vi "bak.W7XBolo2018.vi"(1 "FPGA VI Reference In":refnum<k20>) -> (0 "FPGA VI Reference Out":refnum<k20>)   [LabVIEW 2014]
uses:
  <vilib>/Platform/TimedLoop/XDataNode/timing_clust.ctl
  <vilib>/Platform/TimedLoop/XDataNode/nitl_modes.ctl
  <vilib>/Platform/TimedLoop/XDataNode/wakeup.ctl
  <vilib>/userdefined/High Color/nirio_resource_hc.ctl
  <vilib>/FPGAPlugInAG/PCI-7813R/niLvFpga_Open_PCI-7813R.vi
  <vilib>/Utility/error.llb/Error Cluster From Error Code.vi
  <vilib>/rvi/errors/niLvFpgaAdjustHostInterfaceError.vi
  <vilib>/rvi/interface/common/niFpgaWaitOnOcc.vi
  <vilib>/httpClient/POSTBuffer.vi
  <vilib>/FPGAPlugInAG/PCI-7813R/niLvFpga_Close_PCI-7813R.vi
  <vilib>/rvi/interface/nirviOpenFPGA/nirviOpenFPGA.xnode
  FPGA Bitfiles/W7XBolo2017_FPGATarget_fmain2014_9xlV3GyHFfo.lvbitx
  f_main_2014.vi
  <vilib>/rvi/interface/nirviReadWriteControl/nirviReadWriteControl.xnode
  <vilib>/rvi/interface/nirviMethod/nirviMethod.xnode
  <vilib>/rvi/interface/nirviCloseFPGA/nirviCloseFPGA.xnode
  <vilib>/Platform/TimedLoop/XDataNode/XDataNode.xnode
  <vilib>/Platform/TimedLoop/XDataNode/XDNodeRunTimeDep.lvlib
  <vilib>/Analysis/NI_AALBase.lvlib
  <vilib>/httpClient/LabVIEWHTTPClient.lvlib
  <vilib>/Utility/file.llb/Read From Spreadsheet File (I64).vi
  <vilib>/Utility/file.llb/Read From Spreadsheet File (DBL).vi
  NiFpgaLv.dll
  <vilib>/DAQmx/configure/timing.llb/DAQmx Timing (Sample Clock).vi
  <vilib>/DAQmx/create/channels.llb/DAQmx Create Channel (AO-Voltage-Basic).vi
  <resource>/objmgr/daqmx.rc
  <vilib>/DAQmx/write.llb/DAQmx Write (Analog 1D DBL 1Chan NSamp).vi
  <vilib>/FPGAPlugInAG/PCI-7813R/niLvFpga_AcknowledgeIrq_PCI-7813R.vi
  <vilib>/FPGAPlugInAG/PCI-7813R/niLvFpga_ConfigureFifo_PCI-7813R.vi
  <vilib>/rvi/errors/niLvFpgaMergeErrorWithErrorCode.vi
panel:
  out "DAQ ready":bool
  out "DAQ wait time (should be = TWT":i32=-1
  in  "Pre-start time (ms) of DAQ \nTypically set to 1000 ms":i32=1000
  out "DAQ Timer":dbl
  in  "Tab Control 7":T1(tab)
  in  "Load from file":bool=TRUE
  in  "FreqSelRing":u16(ring) items=["0.8 ms", "1.6 ms", "3.2 ms", "6.4 ms", "12.8 ms", "19.2 ms"]
  in  "SecondFilter":bool=TRUE
  out "SampleTime":sgl=0.0004
  in  "Global or Individual DAC Settings\n\nIf global, dial on the right works.\nIf individual, enabled to either input manually via the array in IRS [Individual Range Settings] or load via file below.":bool caption="Range?"
  in  "DAC Range Setting":u8(knob)=3 scale=0.0..3.0
  in  "No. of Samples:":u32=10000
  out "Measured Time for DAQ [ms]\n \nShould rougly correspond to\nSampleTime * Samples":u32=8048
  in  "DAC settings file location":path=path "C:/LABVIEW/BLVFlo/LABVIEW/BLV/bolo_files/dac_settings.dat"
  in  "Trigger Source":i32(slide)=1 scale=0.0..2.0
  in  "Set Manual Time [ns]":i64=1503619200000000000
  out "Presamples \n(If -1, then no trigger detected)":i32
  in  "Wait-Time until Trigger\npublished on CODA\ntypically 10 s":u32=5000
  out "current epoch time timestamp":timestamp
  out "Number of nanoseconds with offset to 1904":i32
  out "Calibration Time":u32
  out "Countdown Time":u32
  out "Total wait time (TWT)\nTypically 59 s":u32
  in  "time before T1 = T0\nUsusally 60s":i32=60000
  in  "Tau00":dbl[](array[numeric])
  in  "Kappa00":dbl[](array[numeric])
  in  "RB000":dbl[](array[numeric])
  in  "Switch to fixed \nCalibration Values":bool
  in  "Clear all Values \nfrom Beginning":bool
  in  "Cancel Button":bool
  out "Actual Depth":u32=256
  out "T-Start [for Display)\nShould be -1 [s]":sgl=-1.0
  in  "Trigger No Choice\nfrom MDS+ Website\n0 for old\n1 during OP":i32
  in  "Tab Control":T2(tab)
  out "subvi timing":dbl
  out "rand plot sub":cluster{i32, "element":dbl}[](graph)
  in  "channel selection input":i32[][](array[numeric])
  out "kbolott_and_volume":dbl[][](array[numeric])
  in  "Read from file?":bool=TRUE
  in  "Path to kbolott and volume data file":path=path "C:/LABVIEW/BLVFlo/LABVIEW/BLV/bolo_files/kbolott_volume_all.dat"
  in  "Path to channel selection file":path=path "C:/LABVIEW/BLVFlo/LABVIEW/BLV/bolo_files/channel_selection.dat"
  in  "Read Channel Selection from file":bool=TRUE
  out "Channel Selection\nfrom input?":bool
  out "file import":i64[][](array[numeric])
  out "rand plot main":cluster{i32, "element":dbl}[](graph)
  out "sample array":i32[](array[numeric])
  out "cycle #":i32
  out "random array main":dbl[](array[numeric])
  out "rand array sub display":dbl[](array[numeric])
  out "timing average":dbl format="%.2f"
  out "final channel selection":i64[][](array[numeric])
  out "total\ntime":dbl
  out "pick-up cycle":i32
  out "subvi cycle #":dbl
  out "random array sub":dbl[](array[numeric])
  out "final channel\nselection size":i32
  in  "SubVI Test\nwith RAND array and\ntime measurement":bool
  out "Nsample array":i32[](array[numeric])
  out "real time p_rad":cluster{cluster{i32, dbl}[]}[](graph)
  out "RT P_rad":dbl[][](array[numeric])
  out "full power array":dbl[][](array[numeric])
  out "av power array":dbl[](array[numeric])
  out "final P_rad":dbl[](array[numeric])
  out "current P_rad sample":dbl format="%#_13g"
  in  "sample mode":i32(ring)=10123 items=["Finite Samples"=10178, "Continuous Samples"=10123, "Hardware Timed Single Point"=12522]
  in  "RegenMode":i32(ring)=10158 items=["Allow Regeneration"=10097, "Do Not Allow Regeneration"=10158]
  in  "rate of voltage sampling":dbl=100000.0 format="%#_13g"
  out "number of samples written on channel":u32
  in  "Stop Voltage Output":bool
  in  "maximum voltage @ 10MW":dbl=5.0 format="%#_13g"
  out "number of samples per iteration":dbl
  in  "Tab Control 4":enum32{"1 to 64", "65 to 128"}(tab)
  out "Raw 33-64":T3={"Channels 33 - 40"={"tstart"=-1.0, "FPGSampleTime"=0.0007999999797903001, array8x10000[80000 elements]}, "Channels 41 - 48"={"tstart"=-1.0, "FPGSampleTime"=0.0007999999797903001, array8x10000[80000 elements]}, "Channels 49 - 56"={"tstart"=-1.0, "FPGSampleTime"=0.0007999999797903001, array8x10000[80000 elements]}, "Channels 57 - 64"={"tstart"=-1.0, "FPGSampleTime"=0.0007999999797903001, array8x10000[80000 elements]}}
  out "Raw 1-32":T4={"Channels 1- 8"={"tstart"=-1.0, "FPGSampleTime"=0.0007999999797903001, array8x10000[80000 elements]}, "Channels 9 - 16"={"tstart"=-1.0, "FPGSampleTime"=0.0007999999797903001, array8x10000[80000 elements]}, "Channels 17 - 24"={"tstart"=-1.0, "FPGSampleTime"=0.0007999999797903001, array8x10000[80000 elements]}, "Channels 25 - 32"={"tstart"=-1.0, "FPGSampleTime"=0.0007999999797903001, array8x10000[80000 elements]}}
  out "Raw 97 - 128":T5
  out "Raw 65 - 97":T6={"Channels 65 - 71"={"tstart"=-1.0, "FPGSampleTime"=0.0007999999797903001, array8x10000[80000 elements]}, "Channels 73 - 80"={"tstart"=0.0, "FPGSampleTime"=0.0, []}, "Channels 81 - 88"={"tstart"=0.0, "FPGSampleTime"=0.0, []}, "Channels 89- 96"={"tstart"=0.0, "FPGSampleTime"=0.0, []}}
  in  "Tab Control 6":enum32{"1 to 64", "65 to 128"}(tab)=enum."65 to 128"
  out "Pow 33-64":T3
  out "Pow 1-32":T4={"Channels 1- 8"={"tstart"=-1.0, "FPGSampleTime"=0.0007999999797903001, array8x10000[80000 elements]}, "Channels 9 - 16"={"tstart"=-1.0, "FPGSampleTime"=0.0007999999797903001, array8x10000[80000 elements]}, "Channels 17 - 24"={"tstart"=0.0, "FPGSampleTime"=0.0, []}, "Channels 25 - 32"={"tstart"=0.0, "FPGSampleTime"=0.0, []}}
  out "Pow 97 - 128":T5
  out "Pow 65 - 96":T6={"Channels 65 - 71"={"tstart"=-1.0, "FPGSampleTime"=0.0007999999797903001, array8x10000[80000 elements]}, "Channels 73 - 80"={"tstart"=0.0, "FPGSampleTime"=0.0, []}, "Channels 81 - 88"={"tstart"=0.0, "FPGSampleTime"=0.0, []}, "Channels 89- 96"={"tstart"=0.0, "FPGSampleTime"=0.0, []}}
  out "Take file for DAC?":bool
  out "Take Input for DAC?":bool
  out "Range":u8[](array[numeric])
  out "DAC bits (range /1024)":u16[](array[numeric])
  out "full DAC\nfile input":i64[][](array[numeric])
  in  "input DAC settings":i64[](array[numeric])
  out "size(s)":i32
  out "DAC settings":i64[](array[numeric])
  in  "Tab Control 2":T7(tab)
  out "Offset 1-32":T4
  out "Offset 33-64":T3
  out "Offset 65 - 96":T6
  out "Offset 97 - 128":T5
  out "Mean (mV)":dbl[](array[numeric]) format="%10.6f"
  out "Peak to Peak \n      (microV)":dbl[](array[numeric]) format="%10.6f"
  out "StandardDeviation\n        (microV)":dbl[](array[numeric]) format="%10.7f"
  out "RefStatus 65-96":bool[](array[boolean])
  out "RefStatus 33-64":bool[](array[boolean])
  out "RefStatus 1-32":bool[](array[boolean])
  out "RefStatus 97-128":bool[](array[boolean])
  out "MessStatus 1-32":bool[](array[boolean])
  out "MessStatus 33-64":bool[](array[boolean])
  out "MessStatus 97-128":bool[](array[boolean])
  out "MessStatus 65-96":bool[](array[boolean])
  in  "Tab Control 5":T8(tab)
  out "MessCal 17-32":T9
  out "MessCal 1-16":T10
  out "MessCal 49 - 64":T11
  out "MessCal 33 - 49":T12
  out "MessCal 81 - 96":T13
  out "MessCal 65 - 80":T14
  out "MessCal 113 - 128":T15
  out "MessCal 97 - 112":T16
  out "RMESS":dbl[](array[numeric])
  out "KappaM":dbl[](array[numeric]) format="%10.4e"
  out "TauM":dbl[](array[numeric]) format="%10.4f"
  in  "Tab Control 3":T8(tab)=enum."97 to 128"
  out "RefCal 17-32":T9
  out "RefCal 1-16":T10
  out "RefCal 49 - 64":T11
  out "RefCal 33 - 48":T12
  out "RefCal 65 - 80":T14
  out "RefCal 81 - 96":T13
  out "RefCal 113 - 128":T15
  out "RefCal 97 - 112":T16
  out "TauR":dbl[](array[numeric]) caption="TauM" format="%10.4f"
  out "KappaR":dbl[](array[numeric]) format="%10.4e"
  out "RREF":dbl[](array[numeric])
  out "source":string
  out "code":i32
  out "status":bool
  out "Parlog error out":errorcluster
  out "Parlog error out  2":errorcluster
  out "error out":errorcluster
  out "Timed Out 2":bool
  out "Fehler":bool
  out "Fehler READ U+P":bool
  out "FilterTimeOut":bool
  out "result":bool
  out "headers chanDesc":string="HTTP/1.1 201 Created\r\nServer: Apache-Coyote/1.1\r\nLocation: http://archive-webapi.ipp-hgw.mpg.de/Test/raw/W7X/QSB_Bolometry/File_PARLOG/\r\nContent-Type: text/plain\r\nTransfer-Encoding: chunked\r\nDate: Wed, 15 Jul 2015 13:52:20 GMT\r\n\r\n"
  out "body chanDesc":string="Test/raw/W7X/QSB_Bolometry/File_PARLOG/ created."
  in  "chanDescs":T17(array[cluster])=[{"name"="HBCm_U30_01", "active"=1, "physicalQuantity"={"type"="A"}}, {"name"="HBCm_U30_02", "active"=1, "physicalQuantity"={"type"="A"}}, {"name"="HBCm_U30_03", "active"=1, "physicalQuantity"={"type"="A"}}, {"name"="HBCm_U30_04", "active"=1, "physicalQuantity"={"type"="A"}}, {"name"="HBCm_U30_05", "active"=1, "physicalQuantity"={"type"="A"}}, {"name"="HBCm_U30_06", "active"=1, "physicalQuantity"={"type"="A"}}, {"name"="HBCm_U30_07", "active"=1, "physicalQuantity"={"type"="A"}}, {"name"="HBCm_U30_08", "active"=1, "physicalQuantity"={"type"="A"}}, {"name"="HBCm_U30_09", "active"=1, "physicalQuantity"={"type"="A"}}, {"name"="HBCm_U30_10", "active"=1, "physicalQuantity"={"type"="A"}}, {"name"="HBCm_U30_11", "active"=1, "physicalQuantity"={"type"="A"}}, {"name"="HBCm_U30_12", "active"=1, "physicalQuantity"={"type"="A"}}, {"name"="HBCm_U30_013", "active"=1, "physicalQuantity"={"type"="A"}}, {"name"="HBCm_U30_14", "active"=1, "physicalQuantity"={"type"="A"}}, {"name"="HBCm_U30_15", "active"=1, "physicalQuantity"={"type"="A"}}, {"name"="HBCm_U30_16", "active"=1, "physicalQuantity"={"type"="A"}}, {"name"="HBCm_U30_17", "active"=1, "physicalQuantity"={"type"="A"}}, {"name"="HBCm_U30_18", "active"=1, "physicalQuantity"={"type"="A"}}, {"name"="HBCm_U30_19", "active"=1, "physicalQuantity"={"type"="A"}}, {"name"="HBCm_U30_20", "active"=1, "physicalQuantity"={"type"="A"}}, {"name"="HBCm_U30_21", "active"=1, "physicalQuantity"={"type"="A"}}, {"name"="HBCm_U30_22", "active"=1, "physicalQuantity"={"type"="A"}}, {"name"="HBCm_U30_23", "active"=1, "physicalQuantity"={"type"="A"}}, {"name"="HBCm_U30_24", "active"=1, "physicalQuantity"={"type"="A"}}, {"name"="HBCm_U30_25", "active"=1, "physicalQuantity"={"type"="A"}}, {"name"="HBCm_U30_26", "active"=1, "physicalQuantity"={"type"="A"}}, {"name"="HBCm_U30_27", "active"=1, "physicalQuantity"={"type"="A"}}, {"name"="HBCm_U30_28", "active"=1, "physicalQuantity"={"type"="A"}}, {"name"="HBCm_U30_29", "active"=1, "physicalQuantity"={"type"="A"}}, {"name"="HBCm_U30_30", "active"=1, "physicalQuantity"={"type"="A"}}, {"name"="HBCm_U30_31", "active"=1, "physicalQuantity"={"type"="A"}}, {"name"="HBCm_U30_32", "active"=1, "physicalQuantity"={"type"="A"}}, {"name"="VBCm_V21_01", "active"=1, "physicalQuantity"={"type"="A"}}, {"name"="VBCm_V21_02", "active"=1, "physicalQuantity"={"type"="A"}}, {"name"="VBCm_V21_03", "active"=1, "physicalQuantity"={"type"="A"}}, {"name"="VBCm_V21_04", "active"=1, "physicalQuantity"={"type"="A"}}, {"name"="VBCm_V21_05", "active"=1, "physicalQuantity"={"type"="A"}}, {"name"="VBCm_V21_06", "active"=1, "physicalQuantity"={"type"="A"}}, {"name"="VBCm_V21_07", "active"=1, "physicalQuantity"={"type"="A"}}, {"name"="VBCm_V21_08", "active"=1, "physicalQuantity"={"type"="A"}}, {"name"="VBCm_V21_09", "active"=1, "physicalQuantity"={"type"="A"}}, {"name"="VBCm_V21_10", "active"=1, "physicalQuantity"={"type"="A"}}, {"name"="VBCm_V21_11", "active"=1, "physicalQuantity"={"type"="A"}}, {"name"="VBCm_V21_12", "active"=1, "physicalQuantity"={"type"="A"}}, {"name"="VBCm_V21_13", "active"=1, "physicalQuantity"={"type"="A"}}, {"name"="VBCm_V21_14", "active"=1, "physicalQuantity"={"type"="A"}}, {"name"="VBCm_V21_15", "active"=1, "physicalQuantity"={"type"="A"}}, {"name"="VBCm_V21_16", "active"=1, "physicalQuantity"={"type"="A"}}, {"name"="VBCm_V21_17", "active"=1, "physicalQuantity"={"type"="A"}}, {"name"="VBCm_V21_18", "active"=1, "physicalQuantity"={"type"="A"}}, {"name"="VBCm_V21_19", "active"=1, "physicalQuantity"={"type"="A"}}, {"name"="VBCm_V21_20", "active"=1, "physicalQuantity"={"type"="A"}}, {"name"="VBCm_V21_21", "active"=1, "physicalQuantity"={"type"="A"}}, {"name"="VBCm_V21_22", "active"=1, "physicalQuantity"={"type"="A"}}, {"name"="VBCm_V21_23", "active"=1, "physicalQuantity"={"type"="A"}}, {"name"="VBCm_V21_24", "active"=1, "physicalQuantity"={"type"="A"}}, {"name"="VBCm_V21_25", "active"=1, "physicalQuantity"={"type"="A"}}, {"name"="VBCm_V21_26", "active"=1, "physicalQuantity"={"type"="A"}}, {"name"="VBCm_V21_27", "active"=1, "physicalQuantity"={"type"="A"}}, {"name"="VBCm_V21_28", "active"=1, "physicalQuantity"={"type"="A"}}, {"name"="VBCm_V21_29", "active"=1, "physicalQuantity"={"type"="A"}}, {"name"="VBCm_V21_30", "active"=1, "physicalQuantity"={"type"="A"}}, {"name"="VBCm_V21_31", "active"=1, "physicalQuantity"={"type"="A"}}, {"name"="VBCm_V21_32", "active"=1, "physicalQuantity"={"type"="A"}}, {"name"="VBCm_V21_33", "active"=1, "physicalQuantity"={"type"="A"}}, {"name"="VBCm_V21_34", "active"=1, "physicalQuantity"={"type"="A"}}, {"name"="VBCm_V21_35", "active"=1, "physicalQuantity"={"type"="A"}}, {"name"="VBCm_V21_36", "active"=1, "physicalQuantity"={"type"="A"}}, {"name"="VBCm_V21_37", "active"=1, "physicalQuantity"={"type"="A"}}, {"name"="VBCm_V21_38", "active"=1, "physicalQuantity"={"type"="A"}}, {"name"="VBCm_V21_39", "active"=1, "physicalQuantity"={"type"="A"}}, {"name"="VBCm_V21_40", "active"=1, "physicalQuantity"={"type"="A"}}, {"name"="VBCs_V21_01", "active"=1, "physicalQuantity"={"type"="A"}}, {"name"="VBCs_V21_02", "active"=1, "physicalQuantity"={"type"="A"}}, {"name"="VBCs_V21_03", "active"=1, "physicalQuantity"={"type"="A"}}, {"name"="VBCs_V21_04", "active"=1, "physicalQuantity"={"type"="A"}}, {"name"="VBCs_V21_05", "active"=1, "physicalQuantity"={"type"="A"}}, {"name"="VBCs_V21_06", "active"=1, "physicalQuantity"={"type"="A"}}, {"name"="VBCs_V21_07", "active"=1, "physicalQuantity"={"type"="A"}}, {"name"="VBCs_V21_08", "active"=1, "physicalQuantity"={"type"="A"}}, {"name"="HBCs_U30_01", "active"=1, "physicalQuantity"={"type"="A"}}, {"name"="HBCs_U30_02", "active"=1, "physicalQuantity"={"type"="A"}}, {"name"="HBCs_U30_03", "active"=1, "physicalQuantity"={"type"="A"}}, {"name"="HBCs_U30_04", "active"=1, "physicalQuantity"={"type"="A"}}, {"name"="HBCs_U30_05", "active"=1, "physicalQuantity"={"type"="A"}}, {"name"="HBCs_U30_06", "active"=1, "physicalQuantity"={"type"="A"}}, {"name"="HBCs_U30_07", "active"=1, "physicalQuantity"={"type"="A"}}, {"name"="HBCs_U30_08", "active"=1, "physicalQuantity"={"type"="A"}}, {"name"="HBCs_U30_09", "active"=1, "physicalQuantity"={"type"="A"}}, {"name"="HBCs_U30_10", "active"=1, "physicalQuantity"={"type"="A"}}, {"name"="HBCs_U30_11", "active"=1, "physicalQuantity"={"type"="A"}}, {"name"="HBCs_U30_12", "active"=1, "physicalQuantity"={"type"="A"}}, {"name"="HBCs_U30_13", "active"=1, "physicalQuantity"={"type"="A"}}, {"name"="HBCs_U30_14", "active"=1, "physicalQuantity"={"type"="A"}}, {"name"="HBCs_U30_15", "active"=1, "physicalQuantity"={"type"="A"}}, {"name"="HBCs_U30_16", "active"=1, "physicalQuantity"={"type"="A"}}]
  out "error out Cal":errorcluster
  out "parms error out":errorcluster
  in  "stop":bool
  out "Acquired Samples:":u32(slide) scale=-1.0..10000.0
  out "state":string="Wait for Start"
  # "If individual Range DAC Setting is selected, \nthe gain Range is loaded from following file:"
  # "Largest Offset ~ 20 mV\n40 mV Range should work \nfor all channels"
  # "Sample Rate Settings"
  # "FilterSelection"
  # "Set manual time [ns], epoch time"
  # "Get last trigger from http://sv-coda-wsvc-3/last_trigger"
  # "Get UTC Time not working"
  # "WENDELSTEIN - 7-X Bolometer DAQ System                                                                  v1.1.0"
  # "2018 @ P.Hacker"
  # "DAC Range shown for check:"
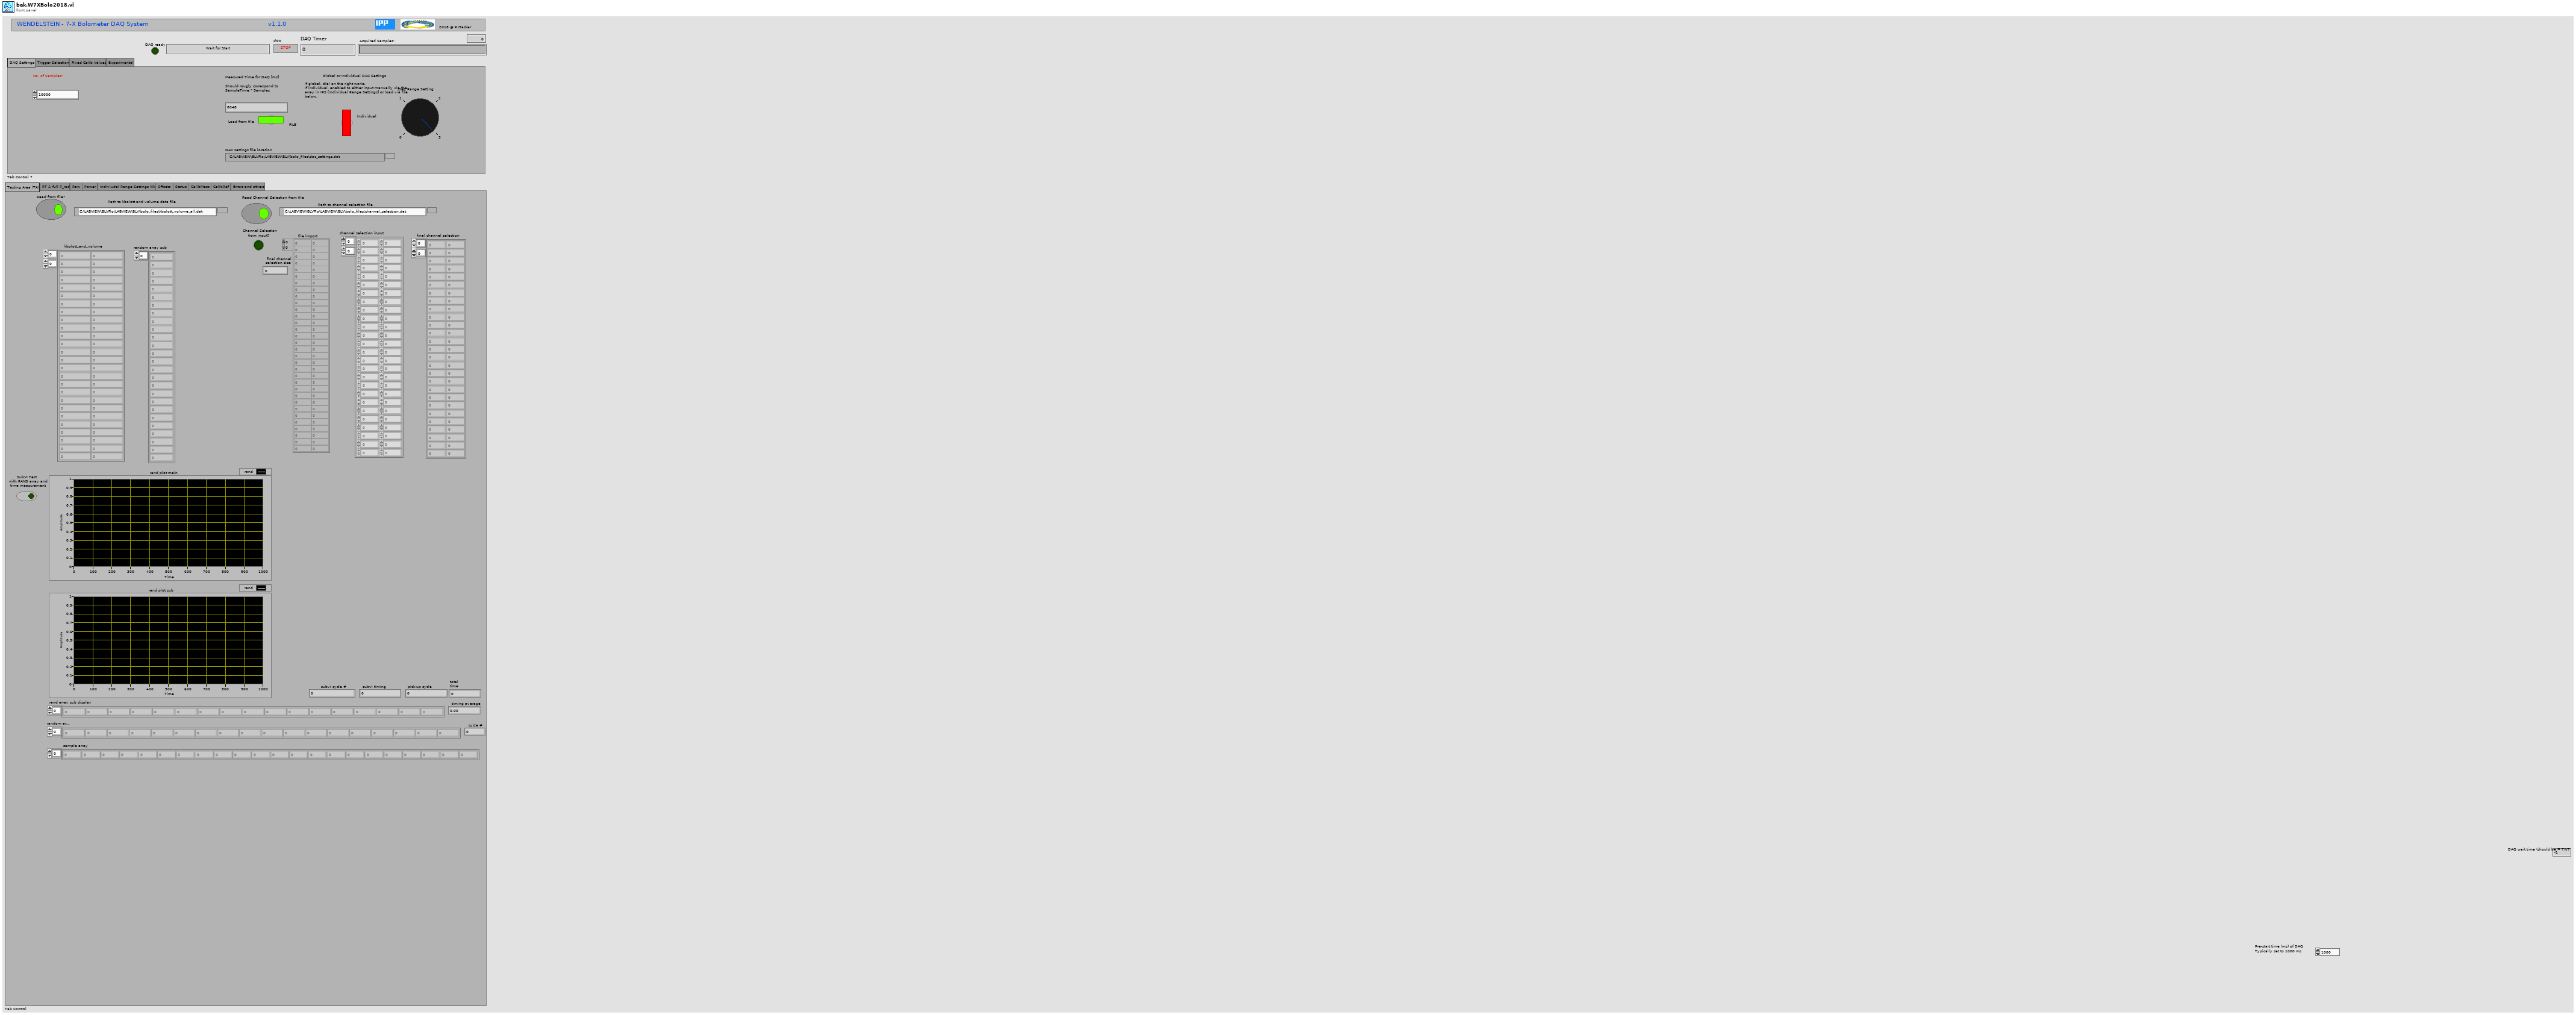
[diagram p1: front panel]
types:
  T1 = enum32{"DAQ Settings", "Trigger Selection", "Fixed Calib Values", "Experimental"}
  T2 = enum32{"Testing Area (TA)", "RT & full P_rad", "Raw", "Power", "Indiviudal Range Settings (IRS)", "Offsets", "Status", "CalibMess", "CalibRef", "Errors and others"}
  T3 = cluster{"Channels 33 - 40":cluster{"tstart":dbl, "FPGSampleTime":dbl, dbl[][]}, "Channels 41 - 48":cluster{"tstart":dbl, "FPGSampleTime":dbl, dbl[][]}, "Channels 49 - 56":cluster{"tstart":dbl, "FPGSampleTime":dbl, dbl[][]}, "Channels 57 - 64":cluster{"tstart":dbl, "FPGSampleTime":dbl, dbl[][]}}
  T4 = cluster{"Channels 1- 8":cluster{"tstart":dbl, "FPGSampleTime":dbl, dbl[][]}, "Channels 9 - 16":cluster{"tstart":dbl, "FPGSampleTime":dbl, dbl[][]}, "Channels 17 - 24":cluster{"tstart":dbl, "FPGSampleTime":dbl, dbl[][]}, "Channels 25 - 32":cluster{"tstart":dbl, "FPGSampleTime":dbl, dbl[][]}}
  T5 = cluster{"Channels 97 - 104":cluster{"tstart":dbl, "FPGSampleTime":dbl, dbl[][]}, "Channels 105 - 112":cluster{"tstart":dbl, "FPGSampleTime":dbl, dbl[][]}, "Channels 113 - 120":cluster{"tstart":dbl, "FPGSampleTime":dbl, dbl[][]}, "Channels 121 - 128":cluster{"tstart":dbl, "FPGSampleTime":dbl, dbl[][]}}
  T6 = cluster{"Channels 65 - 71":cluster{"tstart":dbl, "FPGSampleTime":dbl, dbl[][]}, "Channels 73 - 80":cluster{"tstart":dbl, "FPGSampleTime":dbl, dbl[][]}, "Channels 81 - 88":cluster{"tstart":dbl, "FPGSampleTime":dbl, dbl[][]}, "Channels 89- 96":cluster{"tstart":dbl, "FPGSampleTime":dbl, dbl[][]}}
  T7 = enum32{"1 to 32", "33 to 64", "65 to 96", "97 to128"}
  T8 = enum32{"1 to 32", "33 to 64", "65 to 96", "97 to 128"}
  T9 = cluster{"Channels 17 - 20":cluster{"tstart":sgl, "dt":sgl, "OutArray":dbl[][]}, "Channels 21 - 24":cluster{"tstart":sgl, "dt":sgl, "OutArray":dbl[][]}, "Channels 25 - 28":cluster{"tstart":sgl, "dt":sgl, "OutArray":dbl[][]}, "Channels 29 - 32":cluster{"tstart":sgl, "dt":sgl, "OutArray":dbl[][]}}
  T10 = cluster{"Channels 1- 4":cluster{"tstart":sgl, "dt":sgl, "OutArray":dbl[][]}, "Channels 5 - 8":cluster{"tstart":sgl, "dt":sgl, "OutArray":dbl[][]}, "Channels 9 - 12":cluster{"tstart":sgl, "dt":sgl, "OutArray":dbl[][]}, "Channels 13 - 16":cluster{"tstart":sgl, "dt":sgl, "OutArray":dbl[][]}}
  T11 = cluster{"Channels 49 - 52":cluster{"tstart":sgl, "dt":sgl, "OutArray":dbl[][]}, "Channels 53 - 56":cluster{"tstart":sgl, "dt":sgl, "OutArray":dbl[][]}, "Channels 57 - 60":cluster{"tstart":sgl, "dt":sgl, "OutArray":dbl[][]}, "Channels 61 - 64":cluster{"tstart":sgl, "dt":sgl, "OutArray":dbl[][]}}
  T12 = cluster{"Channels 33 - 36":cluster{"tstart":sgl, "dt":sgl, "OutArray":dbl[][]}, "Channels 37 - 40":cluster{"tstart":sgl, "dt":sgl, "OutArray":dbl[][]}, "Channels 41 - 44":cluster{"tstart":sgl, "dt":sgl, "OutArray":dbl[][]}, "Channels 45 - 48":cluster{"tstart":sgl, "dt":sgl, "OutArray":dbl[][]}}
  T13 = cluster{"Channels 81 - 84":cluster{"tstart":sgl, "dt":sgl, "OutArray":dbl[][]}, "Channels 85 - 88":cluster{"tstart":sgl, "dt":sgl, "OutArray":dbl[][]}, "Channels 89 - 92":cluster{"tstart":sgl, "dt":sgl, "OutArray":dbl[][]}, "Channels 93 - 96":cluster{"tstart":sgl, "dt":sgl, "OutArray":dbl[][]}}
  T14 = cluster{"Channels 65 - 68":cluster{"tstart":sgl, "dt":sgl, "OutArray":dbl[][]}, "Channels 69 - 72":cluster{"tstart":sgl, "dt":sgl, "OutArray":dbl[][]}, "Channels 73 - 76":cluster{"tstart":sgl, "dt":sgl, "OutArray":dbl[][]}, "Channels 77 - 80":cluster{"tstart":sgl, "dt":sgl, "OutArray":dbl[][]}}
  T15 = cluster{"Channels 113 - 116":cluster{"tstart":sgl, "dt":sgl, "OutArray":dbl[][]}, "Channels 117 - 120":cluster{"tstart":sgl, "dt":sgl, "OutArray":dbl[][]}, "Channels 121 - 124":cluster{"tstart":sgl, "dt":sgl, "OutArray":dbl[][]}, "Channels 125 - 128":cluster{"tstart":sgl, "dt":sgl, "OutArray":dbl[][]}}
  T16 = cluster{"Channels 97 - 100":cluster{"tstart":sgl, "dt":sgl, "OutArray":dbl[][]}, "Channels 101 - 104":cluster{"tstart":sgl, "dt":sgl, "OutArray":dbl[][]}, "Channels 104 - 108":cluster{"tstart":sgl, "dt":sgl, "OutArray":dbl[][]}, "Channels 109 - 112":cluster{"tstart":sgl, "dt":sgl, "OutArray":dbl[][]}}
  T17 = cluster{"name":string, "active":i32, "physicalQuantity":cluster{"type":string}}[]
  T18 = cluster{"Nchannel":i16, "ADCbits":i16, "BridgeVoltage (V)":sgl, "ExptSampleFrequency (Hz)":sgl, "CalibSampleFrequency (Hz)":sgl, "CalStep1 (V)":string, "CalStep2 (V)":string, "detector":string}[]
  T19 = cluster{"chanDescs":cluster{"name":string, "active":i32}[]}[]
  T20 = cluster{"tstart":sgl, "dt":sgl, "OutArray":dbl[][]}
  T21 = cluster{"Channels 9 - 12":cluster{"tstart":sgl, "dt":sgl, "OutArray":dbl[][]}, "Channels 9 - 12":cluster{"tstart":sgl, "dt":sgl, "OutArray":dbl[][]}, "Channels 9 - 12":cluster{"tstart":sgl, "dt":sgl, "OutArray":dbl[][]}, "Channels 9 - 12":cluster{"tstart":sgl, "dt":sgl, "OutArray":dbl[][]}}
  T22 = typedef "XDNodeRunTimeDep.lvlib/timing_clust.ctl" = cluster{"Expected End [f-1]":u64, "Actual End [f-1]":u64, "Finished Late? [f-1]":bool, "Expected End [i-1]":u64, "Actual End [i-1]":u64, "Finished Late? [i-1]":bool, "Expected Start [i]":u64, "Actual Start [i]":u64, "Expected Start [f]":u64, "Actual Start [f]":u64, "Source Name":string, "Structure Name":string, "Period":i64, "Deadline":i64, "Offset":i64, "Start":i64, "Priority":i32, "Timeout":i32, "Mode":T23, "Wakeup Reason":T24, "Error":errorcluster, "Source Type":string, "Secondary Source Type":string, "Global End Time":u64, "Global Start Time":u64, "Frame Duration":u64, "Iteration Duration":u64, "Assigned CPU":i32, "I/O Scan Engine Mode":u32}
  T23 = typedef "XDNodeRunTimeDep.lvlib/nitl_modes.ctl" = enum32{"No Change", "Process missed periods, maintain original phase", "Discard missed periods, maintain original phase", "Process missed periods, ignore original phase", "Discard missed periods, ignore original phase"}
  T24 = typedef "XDNodeRunTimeDep.lvlib/wakeup.ctl" = enum32{"Normal", "Aborted", "Asynchronous wakeup", "Timing source error", "Timed loop error", "Timeout"}
  T25 = typedef "nirio_resource_hc.ctl" = tag
  T26 = cluster{"Channels 33 - 40":cluster{"tstart":dbl, "FPGSampleTime":dbl, dbl[][]}, "Channels 41 - 48":cluster{"tstart":dbl, "FPGSampleTime":dbl, dbl[][]}, "Channels 49 - 56":cluster{"tstart":dbl, "FPGSampleTime":dbl, dbl[][]}, "Channels 57 - 58":cluster{"tstart":dbl, "FPGSampleTime":dbl, dbl[][]}}
  T27 = cluster{"Channels 1- 8":cluster{"tstart":sgl, "dt":sgl, "OutArray":dbl[][]}, "Channels 9 - 16":cluster{"tstart":sgl, "dt":sgl, "OutArray":dbl[][]}, "Channels 17 - 24":cluster{"tstart":sgl, "dt":sgl, "OutArray":dbl[][]}, "Channels 25 - 32":cluster{"tstart":sgl, "dt":sgl, "OutArray":dbl[][]}}
  T28 = cluster{"Channels 33 - 40":cluster{"tstart":sgl, "dt":sgl, "OutArray":dbl[][]}, "Channels 41 - 48":cluster{"tstart":sgl, "dt":sgl, "OutArray":dbl[][]}, "Channels 49 - 56":cluster{"tstart":sgl, "dt":sgl, "OutArray":dbl[][]}, "Channels 57 - 58":cluster{"tstart":sgl, "dt":sgl, "OutArray":dbl[][]}}
  T29 = typedef "LabVIEWHTTPClient.lvlib/ClientHandle.ctl" = refnum<k1>
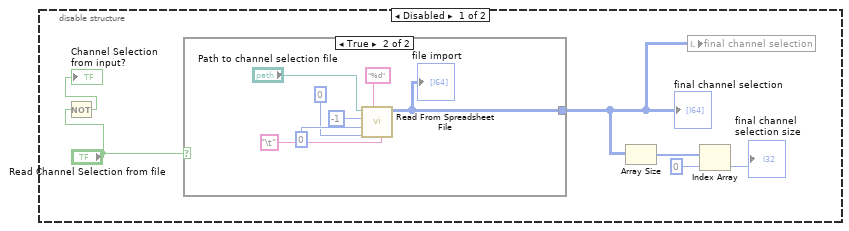
[diagram p5: hidden frame]
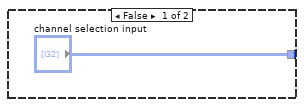
[diagram p6: hidden frame]
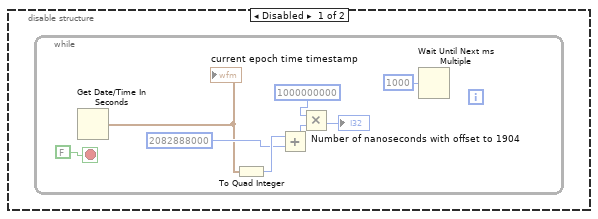
[diagram p7: hidden frame]
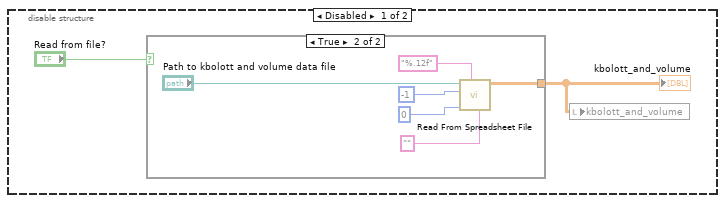
[diagram p8: hidden frame]
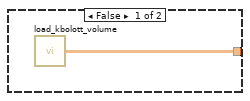
[diagram p9: hidden frame]
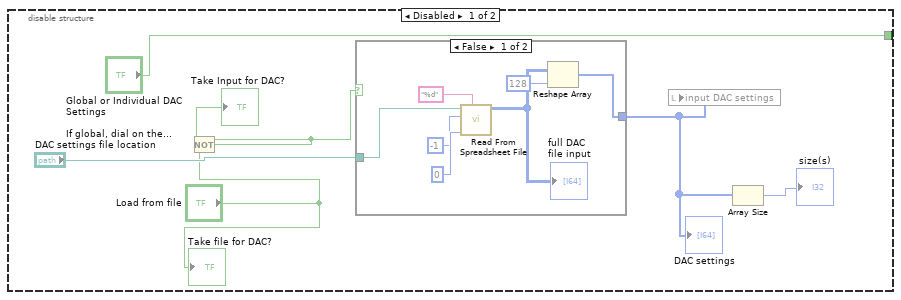
[diagram p10: hidden frame]
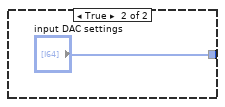
[diagram p11: hidden frame]
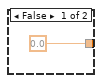
[diagram p14: hidden frame]
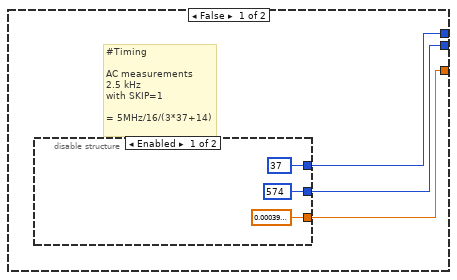
[diagram p17: hidden frame]
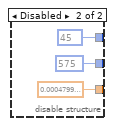
[diagram p18: hidden frame]
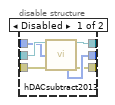
[diagram p19: hidden frame]
diagram:
  w4 = TRUE
  w9 = "W"  # Unit
  w20 = "Float"  # datatype
  w14 = "BoloPower"  # label
  w29 = i64 -1  # Time Array needs to be positive!
  w46 = i64 -1000000000  # Ns per Sec
  w77 = 1 ("sampleCount")
  w78 = 1 ("sampleCount")
  w81 = "s"  # Unit
  w102 = "V"  # Unit
  w106 = "A"  # Unit
  w26 = "A"  # Unit
  w110 = "A"  # Unit
  w117 = 1 ("sampleCount")
  w119 = 1 ("sampleCount")
  w121 = 1 ("sampleCount")
  w76 = 1 ("sampleCount")
  w49 = 1 ("sampleCount")
  w127 = "Float"  # datatype
  w97 = "mV"  # Unit
  w99 = "Offset"
  w133 = "Float"  # datatype
  w94 = "W"  # Unit
  w96 = "RKappa"  # label
  w135 = "Float"  # datatype
  w91 = "Ohms"  # Unit
  w93 = "RRes"  # label
  w137 = "Float"  # datatype
  w88 = "s"  # Unit
  w90 = "RTau"  # label
  w139 = "Float"  # datatype
  w85 = "W"  # Unit
  w87 = "MKappa"  # label
  w141 = "Float"  # datatype
  w84 = "Ohms"  # Unit
  w83 = "MRes"  # label
  w143 = "Float"  # datatype
  w80 = "MTau"  # label
  w50 = 10000 ("dimension size")
  w151 = 10000 ("sampleCount")
  w153 = "Float"  # datatype
  w112 = "A"  # Unit
  w114 = "BoloCalibRefFoilFit"  # label
  w154 = 10000 ("sampleCount")
  w156 = "Float"  # datatype
  w108 = "BoloCalibRefFoilCurrent"  # label
  w157 = 10000 ("sampleCount")
  w159 = "Float"  # datatype
  w6 = "BoloCalibMeasFoilFit"  # label
  w160 = 10000 ("sampleCount")
  w162 = "Float"  # datatype
  w104 = "BoloCalibMeasFoilCurrent"  # label
  w163 = "Float"  # datatype
  w101 = "BoloSignal"  # label
  # "I DONT KNOW ?!"
  # "channel selection routine for RT P_rad estimation"
  # "global switch for DAC settings and input relations, as well as ranges"
  # "import and load the kbolott and volume data for each camera/channel"
  # "time display for manual trigger and time stamp"
  # "SubVI, Reference and timeout test with basic tmp-VI"
  # "<< BoloCalibRefFoilFit <<"
  # "<< BoloCalibMeasFoilCurrent <<"
  # "<< BoloSignal <<"
  # ">> BoloReffFoilCurrent >>"
  # ">> BoloCalibMeasFoilFit >>"
  # ">> power >>"
  # "> power array >"
  # "> voltage array >"
  # "> voltage array >"
  # "> power >"
  # "Negative Sample Time [ns]"
  # "Time array for Bolo Signal"
  # "No of Samples DAQ"
  # "Time array for Bolo Signal"
  # "+ wait Time"
  # "-800000ns for 0.8ms"
  # "Negative Sample Time [ns]"
  # "Here Changed Names"
  # "Time Stamp for JSON Files"
  # "Sample rate for Calibration Arrays\n should be hardwired to calirbation settings"
  # "Sample Rate in [ns]"
  # "Calculated Start Time [ns]"
  # "NSample"
  # "10000"
  # "Initialize Array:\nDimesions Size = NSamples"
  # "Pulselength fixed for 0.4ms sample time and 10000 samples"
  # "NSamples * SampleTime = PulseLength"
  # "Data here is incorrect as well=!"
  # "Sample Time [s]\ncalculated to \nSample Time [ns]"
  # "Creating virtual Time Stamp\nfor Shot and for Calibration (Hardwired to 10000 samples)\nShot is depending on set sample rate"
  # "Index von dem Sample\nals der Trigger empfangen wurde"
  # "T1 Trigger\nkommt hier"
  # "A=> Internal full scale calibration\n8=> Internal zero scale calibration\nC=> System Zero scale Calibration\n2=> Continuous conversion\n\n5V reference\n80 mV scale\nChannel 1 input (voltage at bridge)\nMaster clock disable\n\np.15 7730 manual"
  # "AC 1.25 kHz Frequenz\nSKIP=0"
  n1 = flat-sequence {
    tunnel: [w207] -> w66
    tunnel: ["FPGA VI Reference In"] -> w70
    tunnel: [w208] -> w69
    tunnel: w66 -> [w208]
    frame #0 {
      n2 = Tick Count (ms)() -> (millisecond timer value=w207:u32)
    }
    frame #1 {
      n3 = case shown="True" "Clear all Values \nfrom Beginning" {
        frame False {
        }
        frame True {
          n4 = flat-sequence {
            frame #0 {
              w212 = bool[] [] ("MessStatus 1-32")
              w211 = dbl[] [] ("Kappa00")
              w214 = T20 {"tstart"=0.0, "dt"=0.0, "OutArray"=[]} ("Channels 9 - 12")
              # "Clear Graphs"
              n5 = local write "MessStatus 1-32"(w212) -> ()
              n6 = local write "RefStatus 97-128"(w212) -> ()
              n7 = local write "MessStatus 33-64"(w212) -> ()
              n8 = local write "MessStatus 65-96"(w212) -> ()
              n9 = local write "MessStatus 97-128"(w212) -> ()
              n10 = local write "RefStatus 1-32"(w212) -> ()
              n11 = local write "RefStatus 33-64"(w212) -> ()
              n12 = local write "RefStatus 65-96"(w212) -> ()
              n13 = local write "TauM"(w211) -> ()
              n14 = local write "TauR"(w211) -> ()
              n15 = local write "Tau00"(w211) -> ()
              n16 = local write "RMESS"(w211) -> ()
              n17 = local write "RREF"(w211) -> ()
              n18 = local write "RB000"(w211) -> ()
              n19 = Bundle("Channels 9 - 12"=w214, "Channels 9 - 12"=w214, "Channels 9 - 12"=w214, "Channels 9 - 12"=w214) -> (w213:T21)  [unwired: 1 in]
              n20 = local write "DAC bits (range /1024)"(w211) -> ()
              n21 = local write "MessCal 1-16"(w213) -> ()
              n22 = local write "MessCal 113 - 128"(w213) -> ()
              n23 = local write "MessCal 17-32"(w213) -> ()
              n24 = local write "MessCal 33 - 49"(w213) -> ()
              n25 = local write "Raw 65 - 97"(w213) -> ()
              n26 = local write "MessCal 49 - 64"(w213) -> ()
              n27 = local write "Raw 97 - 128"(w213) -> ()
              n28 = local write "MessCal 65 - 80"(w213) -> ()
              n29 = local write "MessCal 81 - 96"(w213) -> ()
              n30 = local write "MessCal 97 - 112"(w213) -> ()
              n31 = local write "RefCal 1-16"(w213) -> ()
              n32 = local write "RefCal 113 - 128"(w213) -> ()
              n33 = local write "Raw 1-32"(w213) -> ()
              n34 = local write "Raw 33-64"(w213) -> ()
              n35 = local write "RefCal 33 - 48"(w213) -> ()
              n36 = local write "Pow 1-32"(w213) -> ()
              n37 = local write "RefCal 49 - 64"(w213) -> ()
              n38 = local write "Pow 33-64"(w213) -> ()
              n39 = local write "RefCal 65 - 80"(w213) -> ()
              n40 = local write "Offset 1-32"(w213) -> ()
              n41 = local write "RefCal 81 - 96"(w213) -> ()
              n42 = local write "Offset 33-64"(w213) -> ()
              n43 = local write "RefCal 97 - 112"(w213) -> ()
              n44 = local write "Offset 65 - 96"(w213) -> ()
              n45 = local write "Offset 97 - 128"(w213) -> ()
              n46 = local write "Pow 65 - 96"(w213) -> ()
              n47 = local write "RefCal 17-32"(w213) -> ()
              n48 = local write "Pow 97 - 128"(w213) -> ()
              n49 = local write "KappaR"(w211) -> ()
              n50 = local write "Peak to Peak \n      (microV)"(w211) -> ()
              n51 = local write "Mean (mV)"(w211) -> ()
              n52 = local write "Kappa00"(w211) -> ()
              n53 = local write "StandardDeviation\n        (microV)"(w211) -> ()
              n54 = local write "KappaM"(w211) -> ()
              n55 = local write "Range"(w211) -> ()
            }
          }
        }
      }
    }
  }
  n56 = disable-structure shown="Disabled" {
    frame Disabled {
      n57 = case shown="True" "SubVI Test\nwith RAND array and\ntime measurement" {
        frame False {
        }
        frame True {
          n58 = flat-sequence {
            tunnel: [w220] -> w217
            tunnel: [w219] -> w216
            tunnel: w217 -> [w235]
            tunnel: w216 -> [w229]
            frame #0 {
              w219 = 1000 ("x")
              n59 = Initialize Array(0, w219) -> (w224:i32[])
              n60 = for {
                N: w219 -> [_]
                shift-right: [w225] -> w220
                shift-left: w224 -> [w227]
                i -> [w226]
                n61 = Replace Array Subset(array=w227, new element=w226, index=w226) -> (w225:i32[])
              }
              "sample array" <- w220
              n62 = local write "state"("pre-occupying test arrays" ("state")) -> ()
              n63 = Initialize Array(0.0 ("element"), w219) -> (w218:dbl[])
              "random array main" <- w218
              "random array sub" <- w218
              n64 = local write "random array main"(w218) -> ()
              n65 = local write "random array sub"(w218) -> ()
            }
            frame #1 {
              # "testing for array output"
              n66 = call <vilib>:"High Resolution Relative Seconds.vi"() -> ("relative seconds"=w231:dbl)
              n67 = control-ref of="rand array sub display"() -> (w233:refnum<vi>)
              n68 = local read "No. of Samples:"() -> (w228:u32)
              n69 = for {
                N: w228 -> [_]
                i -> [w241]
                n70 = local read "av power array"() -> (w245:dbl[])
                n71 = local read "final P_rad"() -> (w242:dbl[])
                n72 = Random Number (0-1)() -> (number: 0 to 1=w244:dbl)
                n73 = Replace Array Subset(array=w245, new element=w244, index=w241) -> (w243:dbl[])
                n74 = Random Number (0-1)() -> (number: 0 to 1=w240:dbl)
                n75 = Replace Array Subset(array=w242, new element=w240, index=w241) -> (w239:dbl[])
                n76 = local write "av power array"(w243) -> ()
                n77 = local write "final P_rad"(w239) -> ()
                n78 = Wait Until Next ms Multiple(millisecond multiple=u32 50) -> ()  [unwired: 1 out]
              }
              n79 = control-ref of="subvi cycle #"() -> (w230:refnum<vi>)
              n80 = control-ref of="subvi timing"() -> (w232:refnum<vi>)
              n81 = for {
                N: w229 -> [_]
                tunnel: w235 -> [w258]
                i -> [w259]
                n82 = local read "random array main"() -> (w257:dbl[])
                n83 = Wait Until Next ms Multiple(millisecond multiple=10) -> ()  [unwired: 1 out]
                n84 = Random Number (0-1)() -> (number: 0 to 1=w261:dbl)
                n85 = Replace Array Subset(array=w257, new element=w261, index=w259) -> (w256:dbl[])
                n86 = Build Cluster Array(w258, w256) -> (→"rand plot main":cluster{i32, "element":dbl}[])
                n87 = local write "random array main"(w256) -> ()
                "cycle #" <- w259
              }
              n88 = local read "random array sub"() -> (w234:dbl[])
              n89 = control-ref of="rand plot sub"() -> (w236:refnum<vi>)
              n90 = local write "state"("subvi and real time plot" ("state")) -> ()
              n91 = call "test.vi"("length"=w229, "subvi cycle"=w230, "sample array"=w235, "rand array sub"=w234, "subvi timing"=w232, "Graph Refnum"=w236, "start time"=w231, "rand array sub refnum"=w233) -> ()  [unwired: 4 in]
              n92 = while {
                tunnel: w231 -> [w253]
                tunnel: w229 -> [w247]
                i -> [w249]
                stop <- w254 stop-if-true
                n93 = Multiply(x=w247, y=10) -> (x*y=w248:i32)
                n94 = call <vilib>:"High Resolution Relative Seconds.vi"() -> ("relative seconds"=w252:dbl)
                n95 = Greater?(x=w248, y=w249) -> (0:w254:bool)
                n96 = Subtract(x=w252, y=w253) -> (x-y=w251:dbl)
                "total\ntime" <- w251
                n97 = Divide(x=w251, y=w249) -> (x/y=→"timing average":dbl)
                n98 = Wait Until Next ms Multiple(millisecond multiple=1) -> ()  [unwired: 1 out]
                "pick-up cycle" <- w249
              }
            }
          }
        }
      }
    }
    frame Enabled {
    }
  }
  n99 = Not A Number/Path/Refnum?(number/path/refnum=w70) -> (NaN/Path/Refnum?=w1:bool)
  n100 = disable-structure shown="Enabled" {
    frame Enabled {
      n101 = flat-sequence {
        tunnel: "Cancel" ("name (unnamed)") -> [w292]
        tunnel: "Transferred1" ("name (unnamed)") -> [w291]
        tunnel: u32 0 -> [w290]
        tunnel: FALSE -> [w289]
        tunnel: [w288] -> w271
        tunnel: [w287] -> w270
        tunnel: [w286] -> w269
        tunnel: [w285] -> w268
        tunnel: [u32 0] -> w263
        frame #0 {
          n102 = local write "stop"(FALSE ("stop")) -> ()
          n103 = RT FIFO Create(0:w291, 1:w290) -> (8:w285:refnum<k33>, 11:w286:errorcluster)  [unwired: 2 in, 5 out]
          n104 = RT FIFO Create(0:w292, 1:w289) -> (8:w288:refnum<k33>, 11:w287:errorcluster)  [unwired: 3 in, 4 out]
        }
      }
      n105 = node-c288() -> (w277:T22)  [unwired: 1 in, 4 out]
      n106 = timed-loop {
        tunnel: w271 -> [w303]
        tunnel: w270 -> [w302]
        tunnel: w269 -> [w301]
        tunnel: w268 -> [w300]
        shift-right: [w299] -> _
        shift-left: w263 -> [w293]
        tunnel: [w298] -> w265
        tunnel: [w297] -> w264
        tunnel: [w296] -> w267
        tunnel: [w295] -> w266
        timing: w277 -> [_]
        timing-out: [_] -> w276
        stop <- "stop" stop-if-true
        n107 = RT FIFO Read(0:w300, 1:w293, 3:w301) -> (8:w296:refnum<k33>, 9:w299:u32, 11:w295:errorcluster)  [unwired: 3 out]
        n108 = RT FIFO Write(0:w303, 1:"Cancel Button", 3:w302) -> (8:w298:refnum<k33>, 11:w297:errorcluster)  [unwired: 1 in, 3 out]
        "Acquired Samples:" <- w293
      }
      n109 = node-c288(w276) -> ()  [unwired: 1 out]
      n110 = flat-sequence {
        tunnel: w267 -> [w282]
        tunnel: w266 -> [w281]
        tunnel: w265 -> [w280]
        tunnel: w264 -> [w279]
        frame #0 {
          n111 = RT FIFO Delete(0:w282, 3:w281) -> ()  [unwired: 1 in, 1 out]
          n112 = RT FIFO Delete(0:w280, 3:w279) -> ()  [unwired: 1 in, 1 out]
          n113 = local write "stop"(FALSE ("stop")) -> ()
        }
      }
    }
    frame Disabled {
    }
  }
  n114 = disable-structure shown="Enabled" {
    frame Disabled {
      n115 = while {
        stop <- FALSE stop-if-true
        n116 = Get Date/Time In Seconds() -> (seconds since 1Jan1904=w314:timestamp)
        "current epoch time timestamp" <- w314
        n117 = To Quad Integer(1:w314) -> (0:w316:i64)
        n118 = Add(x=w316, y=2082888000) -> (x+y=w310:i64)
        n119 = Multiply(x=1000000000, y=w310) -> (x*y=→"Number of nanoseconds with offset to 1904":i64)
        n120 = Wait Until Next ms Multiple(millisecond multiple=1000) -> ()  [unwired: 1 out]
      }
    }
    frame Enabled {
    }
  }
  n121 = disable-structure shown="Enabled" {
    frame Disabled {
      n122 = case shown="True" "Read from file?" {
        tunnel: [w319 w320] -> w317
        frame False {
          n123 = call "load_kbolott_volume.vi"() -> ("output"=w319:dbl[][])
        }
        frame True {
          n124 = call-poly <vilib>:"Read From Spreadsheet File.vi"("delimiter (\\t)"="" ("delimiter (\\t)"), "format (%.3f)"="%.12f", "max characters/row  (no limit:0)"=0, "number of rows (all:-1)"=-1, "file path (dialog if empty)"="Path to kbolott and volume data file") -> ("all rows"=w320:dbl[][])  [unwired: 2 in, 4 out]
        }
      }
      "kbolott_and_volume" <- w317
      n125 = local write "kbolott_and_volume"(w317) -> ()
    }
    frame Enabled {
    }
  }
  n126 = disable-structure shown="Enabled" {
    disable-tunnel: ["Global or Individual DAC Settings\n\nIf global, dial on the right works.\nIf individual, enabled to either input manually via the array in IRS [Individual Range Settings] or load via file below." _] -> w3
    frame Disabled {
      n127 = Not(x="Load from file") -> (.not. x?=w329:bool)
      "Take Input for DAC?" <- w329
      n128 = case shown="False" w329 {
        tunnel: "DAC settings file location" -> [w338 _]
        tunnel: [w332 "input DAC settings"] -> w326
        frame False {
          n129 = call-poly <vilib>:"Read From Spreadsheet File.vi"("format (%d)"="%d", "max characters/row  (no limit:0)"=0, "number of rows (all:-1)"=-1, "file path (dialog if empty)"=w338) -> ("all rows"=w333:i64[][])  [unwired: 3 in, 4 out]
          "full DAC\nfile input" <- w333
          n130 = Reshape Array(w333, 128 ("dimension size")) -> (w332:i64[])
        }
        frame True {
        }
      }
      "DAC settings" <- w326
      n131 = local write "input DAC settings"(w326) -> ()
      n132 = Array Size(array=w326) -> (size(s)=→"size(s)":i32)
      "Take file for DAC?" <- "Load from file"
    }
    frame Enabled {
    }
  }
  n133 = disable-structure shown="Enabled" {
    frame Disabled {
      n134 = Not(x="Read Channel Selection from file") -> (.not. x?=→"Channel Selection\nfrom input?":bool)
      n135 = case shown="True" "Read Channel Selection from file" {
        tunnel: ["channel selection input" w347] -> w343
        frame False {
        }
        frame True {
          n136 = call-poly <vilib>:"Read From Spreadsheet File.vi"("delimiter (\\t)"="\t" ("delimiter (\\t)"), "format (%d)"="%d", "max characters/row  (no limit:0)"=0, "start of read offset (chars.:0)"=0, "number of rows (all:-1)"=-1, "file path (dialog if empty)"="Path to channel selection file") -> ("all rows"=w347:i64[][])  [unwired: 1 in, 4 out]
          "file import" <- w347
        }
      }
      "final channel selection" <- w343
      n137 = Array Size(array=w343) -> (size(s)=w342:i32[])
      n138 = local write "final channel selection"(w343) -> ()
      n139 = Index Array(array=w342, index=0) -> (element=→"final channel\nselection size":i32)
    }
    frame Enabled {
    }
  }
  n140 = case shown="True" w1 {
    tunnel: [w354 w356] -> w180
    tunnel: [_ w355] -> w179
    tunnel: w70 -> [w354 _]
    frame False {
    }
    frame True {
      n141 = xnode "Open FPGA VI Reference"("resource name"=T25 "RIO0") -> ("FPGA VI Reference Out"=w356:refnum<k20>, "error out"=w355:errorcluster)  [unwired: 1 in]
    }
  }
  "error out" <- w179
  n142 = xnode "Read/Write Control"("FPGA VI Reference In"=w180, "error in"=w179, "cancel"=TRUE ("clrFifo"), "Test"=FALSE) -> ("FPGA VI Reference Out"=w206:refnum<k20>, "error out"=w205:errorcluster)
  n143 = flat-sequence {
    tunnel: w206 -> [w364]
    tunnel: w205 -> [w363]
    tunnel: [w362] -> w204
    tunnel: [w361] -> w203
    frame #0 {
      n144 = Wait (ms)(milliseconds to wait=u32 100) -> ()  [unwired: 1 out]
      n145 = xnode "Invoke Method"("FPGA VI Reference In"=w364, "error in"=w363, "IRQ Number(s)"=i32[] [0, 1, 2, 3]) -> ("FPGA VI Reference Out"=w362:refnum<k20>, "error out"=w361:errorcluster)
      "state" <- "Start (100 ms)" ("state")
    }
  }
  n146 = flat-sequence {
    tunnel: w203 -> [w366]
    tunnel: [w365] -> w199
    tunnel: w204 -> [w367]
    tunnel: [w368] -> w182
    frame #0 {
      n147 = call "hReset2014.vi"("error in"=w366, "FPGA VI Reference In"=w367) -> ("error out"=w365:errorcluster, "FPGA VI Reference Out"=w368:refnum<k20>)  [unwired: 4 in]
      n148 = local write "state"("Reset" ("state")) -> ()
    }
  }
  n149 = call "hFilterReg2014.vi"("error in"=w199, "Filter Modus"=u16 61 ("t"), "Frequenz"=u8 79 ("AC 1kHz Frequenz\nSKIP=0"), "FPGA VI Reference In"=w182) -> ("error out"=w184:errorcluster, "Timed Out"=w193:bool, "FPGA VI Reference Out"=w183:refnum<k20>)  [unwired: 1 in]
  "FilterTimeOut" <- w193
  n150 = call "hModeReg2014.vi"("error in"=w184, "Mode"=u16 41144, "FPGA VI Reference In"=w183) -> ("error out"=w187:errorcluster, "Timeout"=w197:bool, "FPGA VI Reference Out"=w190:refnum<k20>)  [unwired: 2 in]
  n151 = call "hModeReg2014.vi"("error in"=w187, "Mode"=u16 32952, "FPGA VI Reference In"=w190) -> ("error out"=w186:errorcluster, "Timeout"=w198:bool, "FPGA VI Reference Out"=w189:refnum<k20>)  [unwired: 2 in]
  n152 = call "hModeReg2014.vi"("error in"=w186, "Mode"=u16 8376, "FPGA VI Reference In"=w189) -> ("error out"=w195:errorcluster, "Timeout"=w196:bool, "FPGA VI Reference Out"=w194:refnum<k20>)  [unwired: 2 in]
  n153 = Compound Arithmetic op=OR(w197, w198, w196, w193) -> (→"DAQ ready":bool)
  n154 = case shown="False" w4 {
    tunnel: [w396 w911] -> w67
    tunnel: [w395 w910] -> w202
    tunnel: w194 -> [w555 w911]
    tunnel: w195 -> [w554 w910]
    tunnel: [w415 _] -> w22
    tunnel: [w450 _] -> w149
    tunnel: [w445 _] -> w150
    tunnel: [w441 _] -> w147
    tunnel: [w438 _] -> w148
    tunnel: [w393 _] -> w71
    tunnel: [w436 _] -> w132
    tunnel: [w381 _] -> w72
    tunnel: [w435 _] -> w131
    tunnel: [w434 _] -> w130
    tunnel: [w413 _] -> w129
    tunnel: [w417 _] -> w30
    tunnel: w69 -> [w386 _]
    tunnel: [w383 _] -> w23
    tunnel: [w374 _] -> w21
    tunnel: w3 -> [w373 _]
    frame False {
      w456 = 2000
      w469 = u8 125  # Frequenz
      w514 = 0.0008 ("FPGSampleTime")
      w509 = 0.0
      w380 = 40.0  # Rcable
      w549 = 10.0  # Rload
      w568 = sgl 0.0004  # dt
      w569 = sgl 0.0  # tstart
      w572 = sgl 0.0004  # dt
      w573 = sgl 0.0  # tstart
      w577 = sgl 80.0 ("Scale(mV)")
      # "> voltage array >"
      # "> power >"
      # "> voltage array >"
      # "Offset Shift manually disabled because not need for low power discharges"
      # "Absolute Timer [ms] (Now)\n-\nAbsolute Timer [ms] (At Start)\n=\nTime need until start of DAQ"
      # "Startzeit - 14 s"
      # "old time from OP1"
      # "Store raw data"
      # "#Timing \n\nAC measurements\n2.083 kHz\nwith SKIP=1 \n\n= 5MHz/16/(3*45+15)"
      # "#Offset measurement"
      # "#Offset applied"
      # "#Range for measurements"
      # "A=> Internal full scale calibration\n8=> Internal zero scale calibration\nC=> System Zero scale Calibration\n2=> Continuous conversion\n\n2.5V reference\n80 mV scale\nChannel 2 input (voltage at shunt)\nMaster clock disable\n\np.15 7730 manual"
      n155 = local read "DAC settings"() -> (w372:i64[])
      n156 = flat-sequence {
        tunnel: [w715] -> w391
        tunnel: [w714] -> w390
        tunnel: w555 -> [w718]
        tunnel: w554 -> [w717]
        tunnel: w456 -> [w723]
        tunnel: [w722] -> w458
        tunnel: w391 -> [w725]
        tunnel: w390 -> [w724]
        tunnel: [w721] -> w457
        tunnel: [w731] -> w633
        tunnel: [w730] -> w632
        tunnel: [w729] -> w630
        tunnel: w456 -> [w727]
        tunnel: w458 -> [w733]
        tunnel: w457 -> [w732]
        frame #0 {
          n157 = call "hComRegStart2013.vi"("error in"=w717, "FPGA VI Reference In"=w718) -> ("error out"=w714:errorcluster, "Timed Out"=→"Timed Out 2":bool, "FPGA VI Reference Out"=w715:refnum<k20>)  [unwired: 3 in]
          n158 = call "Wait3"("Count(mSec)"=u32 3000) -> ()  [unwired: 1 out]
        }
        frame #1 {
          n159 = call "Wait6"("Count(mSec)"=u32 1000) -> ()  [unwired: 1 out]
          n160 = local write "state"("SyncRun (1000 ms)" ("state")) -> ()
          n161 = call "hSync&StartSampling2013.vi"("error in"=w724, "#Samples"=w723, "FPGA VI Reference In"=w725) -> ("error out"=w722:errorcluster, "FPGA VI Reference Out"=w721:refnum<k20>)  [unwired: 1 in]
        }
        frame #2 {
          n162 = call "hReadChannelsRTDMA2013.vi"("FPGA VI Reference In"=w732, "Nsamples"=w727, "error in"=w733) -> ("FPGA VI Reference Out"=w731:refnum<k20>, "Fehler"=→"Fehler":bool, "RawArray"=w729:i16[][], "error out"=w730:errorcluster)  [unwired: 2 in]
          n163 = local write "state"("ReadOffset" ("state")) -> ()
        }
      }
      n164 = property on="Acquired Samples:" class="Slide (strict)"("Scale.Range:Maximum"=w456) -> ()  [unwired: 2 in, 2 out]
      n165 = call "hSoftReset2013.vi"("error in"=w632, "FPGA VI Reference In"=w633) -> ("error out"=w467:errorcluster, "FPGA VI Reference Out"=w460:refnum<k20>)  [unwired: 4 in]
      n166 = call "Int2Volt2D.vi"("IntegerArray"=w630, "Scale(mV)"=sgl 80.0) -> ("RealArray"=w505:sgl[][])
      n167 = xnode "Read/Write Control"("FPGA VI Reference In"=w460, "error in"=w467, "HIREF"=TRUE) -> ("FPGA VI Reference Out"=w463:refnum<k20>, "error out"=w462:errorcluster)
      n168 = for {
        tunnel: w505 -> [w754] mode=indexing
        tunnel: [w753] -> w502 mode=indexing
        tunnel: [w752] -> w504 mode=indexing
        tunnel: [w751] -> w503 mode=indexing
        n169 = Array Subset(array=w754, index=500, length=1000) -> (w756:sgl[])
        n170 = call <vilib>:"Std Deviation and Variance.vi"("X"=w756, "Weighting (Sample)"=enum16{"Sample", "Population"}."Population") -> ("mean"=w752:dbl, "standard deviation"=w751:dbl)  [unwired: 1 out]
        n171 = Array Max & Min(array=w756) -> (max value=w759:sgl, min value=w760:sgl)  [unwired: 2 out]
        n172 = Subtract(x=w759, y=w760) -> (x-y=w753:sgl)
      }
      n173 = Array Subset(array=w505, index (row)=0, length (row)=64, index (col)=0) -> (w519:sgl[][])  [unwired: 1 in]
      n174 = Array Subset(array=w505, index (row)=64, length (row)=64, index (col)=0) -> (w515:sgl[][])  [unwired: 1 in]
      n175 = call "Visualize_Signals64.vi"("FPGSampleTime"=w514, "tstart"=w509, "Signals"=w519) -> ("plot(Signals) 33-64"=→"Offset 33-64":T26, "plot(Signals) 1-32"=→"Offset 1-32":T4)  [unwired: 7 in]
      n176 = call "Visualize_Signals64.vi"("FPGSampleTime"=w514, "tstart"=w509, "Signals"=w515) -> ("plot(Signals) 33-64"=→"Offset 97 - 128":T26, "plot(Signals) 1-32"=→"Offset 65 - 96":T4)  [unwired: 7 in]
      n177 = call "hFilterReg2014.vi"("error in"=w462, "Filter Modus"=u16 512 ("t"), "Frequenz"=w469, "FPGA VI Reference In"=w463) -> ("error out"=w461:errorcluster, "FPGA VI Reference Out"=w464:refnum<k20>)  [unwired: 1 in, 1 out]
      n178 = call "hModeReg2014.vi"("error in"=w461, "Mode"=u16 41017, "FPGA VI Reference In"=w464) -> ("error out"=w473:errorcluster, "FPGA VI Reference Out"=w472:refnum<k20>)  [unwired: 2 in, 1 out]
      n179 = call "hModeReg2014.vi"("error in"=w473, "Mode"=u16 32825, "FPGA VI Reference In"=w472) -> ("error out"=w470:errorcluster, "FPGA VI Reference Out"=w471:refnum<k20>)  [unwired: 2 in, 1 out]
      n180 = Multiply(x=w504, y=1000.0 ("Scale")) -> (x*y=w417:dbl[])
      "Mean (mV)" <- w417
      n181 = Multiply(x=w503, y=1000000.0 ("Scale")) -> (x*y=→"StandardDeviation\n        (microV)":dbl[])
      n182 = Multiply(x=w502, y=1000000.0 ("Scale")) -> (x*y=→"Peak to Peak \n      (microV)":dbl[])
      n183 = control-ref of="Acquired Samples:"() -> (w627:refnum<vi>)
      n184 = control-ref of="Cancel Button"() -> (w629:refnum<vi>)
      n185 = call "hModeReg2014.vi"("error in"=w470, "Mode"=u16 8249, "FPGA VI Reference In"=w471) -> ("error out"=w465:errorcluster, "FPGA VI Reference Out"=w466:refnum<k20>)  [unwired: 2 in, 1 out]
      n186 = control-ref of="state"() -> (w628:refnum<vi>)
      n187 = call "hCalRT2013.vi"("FPGA VI Reference In"=w466, "cancelbutton"=w629, "state"=w628, "Acquired Samples"=w627, "error in"=w465) -> ("FPGA VI Reference Out"=w552:refnum<k20>, "Ref"=w576:i16[][], "Meas"=w626:i16[][], "error out"=w551:errorcluster)  [unwired: 6 in, 1 out]
      "error out Cal" <- w551
      n188 = call "Int2Volt2D.vi"("IntegerArray"=w576, "Scale(mV)"=w577) -> ("RealArray"=w578:sgl[][])
      n189 = call "Int2Volt2D.vi"("IntegerArray"=w626, "Scale(mV)"=w577) -> ("RealArray"=w379:sgl[][])
      n190 = flat-sequence {
        tunnel: w552 -> [w744]
        tunnel: w551 -> [w742]
        tunnel: [w743] -> w478
        tunnel: [w741] -> w477
        tunnel: [w748] -> w432
        tunnel: [w747] -> w508
        tunnel: w478 -> [w750]
        tunnel: w477 -> [w749]
        frame #0 {
          w738 = FALSE ("RESET")
          n191 = call "Wait"("Count(mSec)"=u16 3000 ("Count(uSec)")) -> ()  [unwired: 1 out]
          n192 = xnode "Read/Write Control"("FPGA VI Reference In"=w744, "error in"=w742, "RLY1"=w738, "RLY2"=w738, "HIREF"=w738, "Sprung0"=w738, "Sprung1"=w738, "ScanID"=u32 0, "Test"="Switch to fixed \nCalibration Values", "RESET"=TRUE) -> ("FPGA VI Reference Out"=w743:refnum<k20>, "error out"=w741:errorcluster)
          n193 = local write "state"("SoftReset (3000 ms)" ("state")) -> ()
        }
        frame #1 {
          n194 = xnode "Read/Write Control"("FPGA VI Reference In"=w750, "error in"=w749, "RESET"=FALSE) -> ("FPGA VI Reference Out"=w747:refnum<k20>, "error out"=w748:errorcluster)
          n195 = call "Wait5"("Count(mSec)"=u16 1000 ("Count(uSec)")) -> ()  [unwired: 1 out]
        }
      }
      n196 = case shown="True" "SecondFilter" {
        tunnel: [w695 w704] -> w383
        tunnel: [w694 w702] -> w455
        tunnel: [w693 w703] -> w454
        frame False {
          # "#Timing \n\nAC measurements\n2.5 kHz\nwith SKIP=1 \n\n= 5MHz/16/(3*37+14)"
          n197 = disable-structure shown="Enabled" {
            disable-tunnel: [u16 574 ("t") u16 575 ("t")] -> w693
            disable-tunnel: [u16 37 ("frequenz") u16 45 ("frequenz")] -> w694
            disable-tunnel: [sgl 0.0004 sgl 0.00048] -> w695
            frame Enabled {
            }
            frame Disabled {
            }
          }
        }
        frame True {
          # "#Timing \n\nAC measurements\n1.25 kHz\nwith SKIP=0 \n\n= 5MHz/16/250"
          n198 = call "FreqSel.vi"("Ring"="FreqSelRing") -> ("Frequency"=w702:u16, "DLY"=w703:u16, "SampleTime"=w704:sgl)  [unwired: 1 out]
        }
      }
      "SampleTime" <- w383
      n199 = xnode "Invoke Method"("FPGA VI Reference In"=w508, "error in"=w432, "Requested Depth"=u32 256) -> ("FPGA VI Reference Out"=w433:refnum<k20>, "error out"=w431:errorcluster, "Actual Depth"=→"Actual Depth":u32)
      n200 = To Unsigned Byte Integer(number=w372) -> (unsigned 8bit integer=w384:u8[])
      "Range" <- w384
      n201 = call "hFilterReg2014.vi"("error in"=w431, "Filter Modus"=w454, "Frequenz"=w455, "FPGA VI Reference In"=w433) -> ("error out"=w567:errorcluster, "FPGA VI Reference Out"=w566:refnum<k20>)  [unwired: 1 in, 1 out]
      n202 = case shown="True" w373 {
        tunnel: w567 -> [w879 w895]
        tunnel: w566 -> [w880 w894]
        tunnel: [w874 w893] -> w506
        tunnel: [w877 w885] -> w507
        tunnel: u16 41096 -> [w872 w884]
        tunnel: u16 49288 -> [_ w886]
        tunnel: u16 8328 -> [w873 w882]
        tunnel: w384 -> [w871 _]
        tunnel: u16 32904 -> [w869 w883]
        frame False {
          # "MIddle Previously connected xC088 not to x8088"
          n203 = call "hModeRegRange2013.vi"("error in"=w879, "RangeArray"=w871, "Mode"=w872, "FPGA VI Reference In"=w880) -> ("error out"=w876:errorcluster, "FPGA VI Reference Out"=w878:refnum<k20>)  [unwired: 1 in, 1 out]
          n204 = call "hModeRegRange2013.vi"("error in"=w876, "RangeArray"=w871, "Mode"=w869, "FPGA VI Reference In"=w878) -> ("error out"=w875:errorcluster, "FPGA VI Reference Out"=w870:refnum<k20>)  [unwired: 1 in, 1 out]
          n205 = call "hModeRegRange2013.vi"("error in"=w875, "RangeArray"=w871, "Mode"=w873, "FPGA VI Reference In"=w870) -> ("error out"=w874:errorcluster, "FPGA VI Reference Out"=w877:refnum<k20>)  [unwired: 1 in, 1 out]
        }
        frame True {
          n206 = call "hModeReg2014.vi"("error in"=w895, "Range"="DAC Range Setting", "Mode"=w884, "FPGA VI Reference In"=w894) -> ("error out"=w891:errorcluster, "FPGA VI Reference Out"=w892:refnum<k20>)  [unwired: 1 in, 1 out]
          n207 = call "hModeReg2014.vi"("error in"=w891, "Range"="DAC Range Setting", "Mode"=w883, "FPGA VI Reference In"=w892) -> ("error out"=w889:errorcluster, "FPGA VI Reference Out"=w890:refnum<k20>)  [unwired: 1 in, 1 out]
          n208 = disable-structure shown="Enabled" {
            disable-tunnel: w890 -> [w901 w903]
            disable-tunnel: w889 -> [w900 w902]
            disable-tunnel: [w899 w903] -> w888
            disable-tunnel: [w898 w902] -> w887
            disable-tunnel: w886 -> [w897 _]
            disable-tunnel: "DAC Range Setting" -> [w896 _]
            frame Disabled {
              n209 = call "hModeReg2014.vi"("error in"=w900, "Range"=w896, "Mode"=w897, "FPGA VI Reference In"=w901) -> ("error out"=w898:errorcluster, "FPGA VI Reference Out"=w899:refnum<k20>)  [unwired: 1 in, 1 out]
            }
            frame Enabled {
            }
          }
          n210 = call "hModeReg2014.vi"("error in"=w887, "Range"="DAC Range Setting", "Mode"=w882, "FPGA VI Reference In"=w888) -> ("error out"=w893:errorcluster, "FPGA VI Reference Out"=w885:refnum<k20>)  [unwired: 1 in, 1 out]
        }
      }
      n211 = Scale By Power Of 2(n=w384, x=sgl 10.0 ("Scale(mV)")) -> (x*2^n=w385:sgl[])
      n212 = disable-structure shown="Enabled" {
        disable-tunnel: w507 -> [w711 w712]
        disable-tunnel: w506 -> [w710 w713]
        disable-tunnel: w384 -> [w709 _]
        disable-tunnel: [w708 _] -> w485
        disable-tunnel: [w707 w712] -> w480
        disable-tunnel: [w706 w713] -> w426
        frame Disabled {
          n213 = call "hDACsubtract2013.vi"("FPGA VI Reference In"=w711, "Ranges"=w709, "error in"=w710) -> ("FPGA VI Reference Out"=w707:refnum<k20>, "DACbits"=w708:u16[], "error out"=w706:errorcluster)  [unwired: 10 in]
        }
        frame Enabled {
        }
      }
      n214 = Subtract(x=w485, y=u16 1024 ("NSample")) -> (x-y=→"DAC bits (range /1024)":u16[])
      n215 = property on="Acquired Samples:" class="Slide (strict)"(error in=w426, "Scale.Range:Maximum"="No. of Samples:") -> (error out=w425:errorcluster)  [unwired: 1 in, 1 out]
      n216 = flat-sequence {
        tunnel: w425 -> [w763]
        tunnel: w480 -> [w765]
        tunnel: [w764] -> w428
        tunnel: [w762] -> w427
        tunnel: w428 -> [w779]
        tunnel: [w779] -> w422
        tunnel: w427 -> [w778]
        tunnel: [w778] -> w420
        tunnel: w386 -> [w772]
        tunnel: w422 -> [w788]
        tunnel: [w787] -> w421
        tunnel: w420 -> [w786]
        tunnel: [w785] -> w419
        tunnel: "No. of Samples:" -> [w784]
        tunnel: w421 -> [w790]
        tunnel: w419 -> [w791]
        tunnel: w386 -> [w792]
        tunnel: [w790] -> w410
        tunnel: [w791] -> w409
        tunnel: w410 -> [w805]
        tunnel: w409 -> [w804]
        tunnel: [w805] -> w408
        tunnel: [w804] -> w407
        tunnel: [w803] -> w406
        tunnel: w408 -> [w824]
        tunnel: w407 -> [w825]
        tunnel: w406 -> [w819]
        tunnel: "No. of Samples:" -> [w823]
        tunnel: w382 -> [w822]
        tunnel: w405 -> [w813]
        tunnel: w404 -> [w821]
        tunnel: w385 -> [w820]
        tunnel: [w818] -> w403
        tunnel: [w819] -> w402
        tunnel: [w817] -> w401
        tunnel: [w816] -> w400
        tunnel: [w815] -> w399
        tunnel: [w814] -> w398
        tunnel: w371 -> [w812]
        tunnel: w370 -> [w811]
        tunnel: [w864] -> w395
        tunnel: [w865] -> w378
        tunnel: [w866] -> w377
        tunnel: [w867] -> w396
        tunnel: [w868] -> w482
        tunnel: w402 -> [w868]
        tunnel: w401 -> [w867]
        tunnel: w400 -> [w866]
        tunnel: w399 -> [w865]
        tunnel: w398 -> [w864]
        tunnel: [w862] -> w397
        frame #0 {
          n217 = call "Wait4"("Count(mSec)"=u32 1000) -> ()  [unwired: 1 out]
          n218 = local write "state"("Calibration Done" ("state")) -> ()
          n219 = call "hComRegStart2013.vi"("error in"=w763, "FPGA VI Reference In"=w765) -> ("error out"=w762:errorcluster, "FPGA VI Reference Out"=w764:refnum<k20>)  [unwired: 3 in, 1 out]
        }
        frame #1 {
          (unwired) 15000  # fixed -15sec for T0
          n220 = Subtract(x="time before T1 = T0\nUsusally 60s", y="Pre-start time (ms) of DAQ \nTypically set to 1000 ms") -> (x-y=w768:i32)
          "Total wait time (TWT)\nTypically 59 s" <- w768
          n221 = Add(x=w772, y=w768) -> (x+y=w773:u32)
          n222 = Tick Count (ms)() -> (millisecond timer value=w775:u32)
          n223 = local write "state"("Countdown Timer" ("state")) -> ()
          n224 = Subtract(x=w773, y=w775) -> (x-y=w767:u32)
          "Calibration Time" <- w767
          n225 = Subtract(x=w767, y=u32 50) -> (x-y=w769:u32)
          "Countdown Time" <- w769
          n226 = Add(x=w775, y=w769) -> (x+y=w776:u32)
          n227 = while {
            tunnel: w776 -> [w782]
            stop <- w783 continue-if-true
            n228 = Tick Count (ms)() -> (millisecond timer value=w781:u32)
            n229 = Subtract(x=w782, y=w781) -> (x-y=w780:u32)
            "DAQ Timer" <- w780
            n230 = Greater?(x=w782, y=w781) -> (0:w783:bool)
            n231 = local write "DAQ Timer"(w780) -> ()
          }
        }
        frame #2 {
          # "takes 50 ms"
          n232 = call "hSync&StartSampling2013.vi"("error in"=w786, "#Samples"=w784, "FPGA VI Reference In"=w788) -> ("error out"=w785:errorcluster, "FPGA VI Reference Out"=w787:refnum<k20>)  [unwired: 1 in]
        }
        frame #3 {
          n233 = disable-structure shown="Disabled" {
            frame Disabled {
              # "pre-allocation of the sample and signal arrays from the subroutine of measurement"
              # "make sample array that is used in the real time P_rad plot"
              n234 = local read "No. of Samples:"() -> (w799:u32)
              n235 = Initialize Array(0, w799) -> (w796:i32[])
              "Nsample array" <- w796
              n236 = Initialize Array(0.0, w799) -> (w798:dbl[])
              n237 = local write "Nsample array"(w796) -> ()
              n238 = local write "final P_rad"(w798) -> ()
              n239 = local write "av power array"(w798) -> ()
              n240 = for {
                N: w799 -> [_]
                i -> [w801]
                n241 = local read "Nsample array"() -> (w802:i32[])
                n242 = Replace Array Subset(array=w802, new element=w801, index=w801) -> (w800:i32[])
                n243 = local write "Nsample array"(w800) -> ()
              }
            }
            frame Enabled {
            }
          }
          n244 = Tick Count (ms)() -> (millisecond timer value=w793:u32)
          n245 = Subtract(x=w793, y=w792) -> (x-y=→"DAQ wait time (should be = TWT":u32)
          n246 = local write "state"("SyncRun" ("state")) -> ()
        }
        frame #4 {
          n247 = call "Tick Count"() -> ("Tick Count(mSec)"=w803:u32)
        }
        frame #5 {
          # "display acquired arrays from measurement"
          n248 = disable-structure shown="Disabled" {
            frame Disabled {
              n249 = while {
                stop <- FALSE stop-if-true
                n250 = local read "av power array"() -> (w829:dbl[])
                n251 = local read "Nsample array"() -> (w832:i32[])
                n252 = local read "final P_rad"() -> (w830:dbl[])
                n253 = Build Cluster Array(w832, w830) -> (w833:cluster{i32, "element":dbl}[])
                n254 = Build Cluster Array(w832, w829) -> (w831:cluster{i32, "element":dbl}[])
                n255 = Build Cluster Array(w833, w831) -> (→"real time p_rad":cluster{cluster{i32, "element":dbl}[]}[])
                n256 = Wait Until Next ms Multiple(millisecond multiple=u32 1 ("milliseconds to wait")) -> ()  [unwired: 1 out]
              }
            }
            frame Enabled {
            }
          }
          n257 = control-ref of="RT P_rad"() -> (w810:refnum<vi>)
          n258 = control-ref of="full power array"() -> (w809:refnum<vi>)
          n259 = control-ref of="final P_rad"() -> (w808:refnum<vi>)
          n260 = control-ref of="av power array"() -> (w807:refnum<vi>)
          n261 = control-ref of="current P_rad sample"() -> (w806:refnum<vi>)
          n262 = local write "state"("Acquiring Data..." ("state")) -> ()
          n263 = disable-structure shown="Enabled" {
            disable-tunnel: w825 -> [w853 w860]
            disable-tunnel: w824 -> [w852 w861]
            disable-tunnel: w823 -> [w851 w859]
            disable-tunnel: [w850 w858] -> w817
            disable-tunnel: [w849 w857] -> w814
            disable-tunnel: [w848 _] -> w818
            disable-tunnel: w821 -> [w847 _]
            disable-tunnel: w813 -> [w846 _]
            disable-tunnel: [w845 _] -> w816
            disable-tunnel: [w844 w855] -> w815
            disable-tunnel: w822 -> [w843 _]
            disable-tunnel: w820 -> [w842 _]
            disable-tunnel: w812 -> [w841 _]
            disable-tunnel: w811 -> [w840 _]
            disable-tunnel: w810 -> [w838 _]
            disable-tunnel: w809 -> [w839 _]
            disable-tunnel: w808 -> [w837 _]
            disable-tunnel: w807 -> [w836 _]
            disable-tunnel: w806 -> [w835 _]
            frame Enabled {
              n264 = call "hReadChannels-UandP-2013.vi"("FPGA VI Reference In"=w852, "RT P_rad reference"=w838, "final channel selection"=w840, "kbolott_and_volume"=w841, "Nsamples"=w851, "full power array"=w839, "error in"=w853, "Tau/dt"=w843, "Scale(mV)"=w842, "av power array"=w836, "final P_rad"=w837, "RawScal"=w846, "SumScal"=w847, "current P_rad sample"=w835) -> ("Fehler"=w848:bool, "FPGA VI Reference Out"=w850:refnum<k20>, "PowerArray"=w845:sgl[][], "RawArray"=w844:sgl[][], "error out"=w849:errorcluster)  [unwired: 9 in]
            }
            frame Disabled {
              n265 = call "hReadChannelsRTDMA2013.vi"("FPGA VI Reference In"=w861, "Nsamples"=w859, "error in"=w860) -> ("FPGA VI Reference Out"=w858:refnum<k20>, "RawArray"=w856:i16[][], "error out"=w857:errorcluster)  [unwired: 2 in, 1 out]
              n266 = call "Int2Volt2D.vi"("IntegerArray"=w856, "Scale(mV)"=sgl 80.0) -> ("RealArray"=w855:sgl[][])
            }
          }
        }
        frame #6 {
          n267 = local write "state"("Acquiring done" ("state")) -> ()
          n268 = call "Tick Count2"() -> ("Tick Count(mSec)"=w862:u32)
        }
      }
      n269 = disable-structure shown="Disabled" {
        frame Disabled {
          w639 = u16 0 items=["OK message + warnings"]
          w634 = tag "Dev1/ai0"  # DAQmx Physical Channel
          # "voltage loop until halt"
          # "channel prepartions with larger array for busyness"
          # "sampling rate and mode to continuous"
          # "channel preselection for output AO"
          # "number of samples to write until renewal"
          # "rate of sampling"
          # "5 milliseconds"
          n270 = call-poly <vilib>:"DAQmx Create Virtual Channel.vi"("maximum value"="maximum voltage @ 10MW", "minimum value"=0.0, "physical channels"=w634) -> ("task out"=w642:refnum<k21>, "error out"=w643:errorcluster)  [unwired: 11 in]
          n271 = property class="DAQmx Write"(reference=w642, error in=w643, "RegenMode"="RegenMode") -> (reference out=w644:refnum<k21>, error out=w646:errorcluster)
          n272 = call-poly <vilib>:"DAQmx Timing.vi"("task/channels in"=w644, "sample mode"="sample mode", "rate"="rate of voltage sampling", "error in"=w646) -> ("task out"=w647:refnum<k21>, "error out"=w649:errorcluster)  [unwired: 10 in]
          n273 = local read "rate of voltage sampling"() -> (w652:dbl)
          n274 = Multiply(x=0.005, y=w652) -> (x*y=w658:dbl)
          n275 = Round To Nearest(number=w658) -> (nearest integer value=w660:dbl)
          "number of samples per iteration" <- w660
          n276 = Multiply(x=w660, y=2.0) -> (x*y=w661:dbl)
          n277 = Initialize Array(0.0 ("element"), w661) -> (w650:dbl[])
          n278 = call-poly <vilib>:"DAQmx Write.vi"("task/channels in"=w647, "data"=w650, "error in"=w649) -> ("task out"=w653:refnum<k21>, "number of samples written per channel"=→"number of samples written on channel":u32, "error out"=w654:errorcluster)  [unwired: 10 in]
          n279 = call <vilib>:"DAQmx Start Task.vi"("task/channels in"=w653, "error in"=w654) -> ("task out"=w656:refnum<k21>, "error out"=w657:errorcluster)  [unwired: 12 in]
          n280 = while {
            tunnel: w657 -> [w677]
            tunnel: [w667] -> w637
            tunnel: w656 -> [w678]
            tunnel: [w676] -> w636
            stop <- w663 stop-if-true
            # "actually writing smaller data"
            n281 = local read "number of samples per iteration"() -> (w672:dbl)
            n282 = local read "state"() -> (w669:string)
            n283 = local read "state"() -> (w675:string)
            n284 = Equal?(x=w675, y="Acquiring Data...") -> (x = y?=w673:bool)
            n285 = case shown="True" w673 {
              tunnel: [0.0 w680] -> w671
              frame False {
              }
              frame True {
                n286 = local read "current P_rad sample"() -> (w681:dbl)
                n287 = Divide(x=w681, y=2.0) -> (x/y=w680:dbl)
              }
            }
            n288 = Initialize Array(w671, w672) -> (w670:dbl[])
            n289 = call-poly <vilib>:"DAQmx Write.vi"("task/channels in"=w678, "data"=w670, "error in"=w677) -> ("task out"=w676:refnum<k21>, "error out"=w667:errorcluster)  [unwired: 10 in, 1 out]
            n290 = Equal?(x=w669, y="Acquiring done" ("state")) -> (x = y?=w665:bool)
            n291 = Unbundle(w667) -> ("status"=w666:bool)  [unwired: 2 out]
            n292 = Compound Arithmetic op=OR(w666, w665, "Stop Voltage Output") -> (w663:bool)
          }
          n293 = call <vilib>:"DAQmx Clear Task.vi"("task in"=w636, "error in"=w637) -> ("error out"=w638:errorcluster)  [unwired: 13 in]
          n294 = call <vilib>:"Simple Error Handler.vi"("type of dialog (OK msg:1)"=w639, "error in (no error)"=w638) -> ()  [unwired: 3 in, 5 out]
        }
        frame Enabled {
        }
      }
      n295 = local read "Switch to fixed \nCalibration Values"() -> (w565:bool)
      n296 = Divide(x=w379, y=w549) -> (x/y=w442:dbl[][])
      n297 = Add(x=w380, y=w549) -> (x+y=w548:dbl)
      n298 = call "CalFaktor-128.vi"("CalCurrent(t)"=w442, "Rload"=w549, "Rcable"=w380) -> ("FitData"=w437:dbl[][], "Kappa"=w393:dbl[], "Tau"=w381:dbl[], "RB01"=w436:dbl[])  [unwired: 1 out]
      "KappaM" <- w393
      n299 = Array Subset(array=w442, index (row)=0 ("index"), length (row)=128 ("length")) -> (w441:dbl[][])  [unwired: 2 in]
      n300 = case shown="True" w565 {
        tunnel: [w905 "RB000"] -> w550
        tunnel: [w904 "Kappa00"] -> w545
        tunnel: [w906 "Tau00"] -> w382
        tunnel: w381 -> [w906 _]
        tunnel: w436 -> [w905 _]
        tunnel: w393 -> [w904 _]
        frame False {
        }
        frame True {
        }
      }
      n301 = Array Subset(array=w437, index (row)=0 ("index"), length (row)=128 ("length")) -> (w438:dbl[][])  [unwired: 2 in]
      n302 = call "Arraylimit128.vi"("LowerLimit"=400.0, "Array Input"=w436, "UpperLimit"=2000.0) -> ("BoolArray"=w618:bool[], "ArrayOutput"=w392:dbl[])
      "RMESS" <- w392
      n303 = call "Arraylimit128.vi"("LowerLimit"=2e-05, "Array Input"=w393, "UpperLimit"=0.002) -> ("BoolArray"=w620:bool[])  [unwired: 1 out]
      n304 = call "Arraylimit128.vi"("LowerLimit"=0.001, "Array Input"=w381, "UpperLimit"=0.8) -> ("BoolArray"=w619:bool[], "ArrayOutput"=w394:dbl[])
      "TauM" <- w394
      n305 = call "Cal(SubVI)-2013.vi"("Array"=w442, "dt"=w572, "StartChan"=0 ("ChanStart"), "tstart"=w573, "FitData"=w437) -> ("plot(Signals) 1-32"=→"MessCal 1-16":T27, "plot(Signals) 33-64"=→"MessCal 17-32":T28)  [unwired: 9 in]
      n306 = call "Cal(SubVI)-2013.vi"("Array"=w442, "dt"=w572, "StartChan"=64 ("ChanStart"), "tstart"=w573, "FitData"=w437) -> ("plot(Signals) 1-32"=→"MessCal 65 - 80":T27, "plot(Signals) 33-64"=→"MessCal 81 - 96":T28)  [unwired: 9 in]
      n307 = call "Cal(SubVI)-2013.vi"("Array"=w442, "dt"=w572, "StartChan"=96 ("ChanStart"), "tstart"=w573, "FitData"=w437) -> ("plot(Signals) 1-32"=→"MessCal 97 - 112":T27, "plot(Signals) 33-64"=→"MessCal 113 - 128":T28)  [unwired: 9 in]
      n308 = call "Cal(SubVI)-2013.vi"("Array"=w442, "dt"=w572, "StartChan"=32 ("ChanStart"), "tstart"=w573, "FitData"=w437) -> ("plot(Signals) 1-32"=→"MessCal 33 - 49":T27, "plot(Signals) 33-64"=→"MessCal 49 - 64":T28)  [unwired: 9 in]
      n309 = Compound Arithmetic op=OR(w620, w619, w618) -> (w603:bool[])
      n310 = Multiply(x=w548, y=2.0) -> (x*y=w546:dbl)
      n311 = call "U2PCoeff.vi"("Numeric"=w546, "Kappa00"=w545, "RB000"=w550) -> ("Array"=w405:dbl[], "Array 2"=w404:dbl[])
      n312 = Array Subset(array=w603, index=32, length=32) -> (→"MessStatus 33-64":bool[])
      n313 = Array Subset(array=w603, index=64, length=32) -> (→"MessStatus 65-96":bool[])
      n314 = Array Subset(array=w603, index=96, length=32) -> (→"MessStatus 97-128":bool[])
      n315 = Array Subset(array=w603, index=0, length=32) -> (→"MessStatus 1-32":bool[])
      n316 = local read "kbolott_and_volume"() -> (w371:dbl[][])
      n317 = local read "final channel selection"() -> (w370:i64[][])
      n318 = local read "Pre-start time (ms) of DAQ \nTypically set to 1000 ms"() -> (w424:i32)
      n319 = Divide(x=w578, y=w549) -> (x/y=w451:dbl[][])
      n320 = call "CalFaktor-128.vi"("CalCurrent(t)"=w451, "Rload"=w549, "Rcable"=w380) -> ("FitData"=w387:dbl[][], "Kappa"=w413:dbl[], "Tau"=w434:dbl[], "RB01"=w435:dbl[])  [unwired: 1 out]
      "KappaR" <- w413
      n321 = Array Subset(array=w451, index (row)=0 ("index"), length (row)=128 ("length")) -> (w450:dbl[][])  [unwired: 2 in]
      n322 = Array Subset(array=w387, index (row)=0 ("index"), length (row)=128 ("length")) -> (w445:dbl[][])  [unwired: 2 in]
      n323 = call "Arraylimit128.vi"("LowerLimit"=400.0, "Array Input"=w435, "UpperLimit"=2000.0) -> ("BoolArray"=w587:bool[], "ArrayOutput"=w412:dbl[])
      "RREF" <- w412
      n324 = call "Arraylimit128.vi"("LowerLimit"=2e-05, "Array Input"=w413, "UpperLimit"=0.002) -> ("BoolArray"=w585:bool[])  [unwired: 1 out]
      n325 = call "Arraylimit128.vi"("LowerLimit"=0.001, "Array Input"=w434, "UpperLimit"=0.8) -> ("BoolArray"=w586:bool[], "ArrayOutput"=w414:dbl[])
      "TauR" <- w414
      n326 = Subtract(x=w397, y=w482) -> (x-y=→"Measured Time for DAQ [ms]\n \nShould rougly correspond to\nSampleTime * Samples":u32)
      n327 = call "Cal(SubVI)-2013.vi"("Array"=w451, "dt"=w568, "StartChan"=0 ("ChanStart"), "tstart"=w569, "FitData"=w387) -> ("plot(Signals) 1-32"=→"RefCal 1-16":T27, "plot(Signals) 33-64"=→"RefCal 17-32":T28)  [unwired: 9 in]
      n328 = call "Cal(SubVI)-2013.vi"("Array"=w451, "dt"=w568, "StartChan"=32 ("ChanStart"), "tstart"=w569, "FitData"=w387) -> ("plot(Signals) 1-32"=→"RefCal 33 - 48":T27, "plot(Signals) 33-64"=→"RefCal 49 - 64":T28)  [unwired: 9 in]
      n329 = call "Cal(SubVI)-2013.vi"("Array"=w451, "dt"=w568, "StartChan"=96 ("ChanStart"), "tstart"=w569, "FitData"=w387) -> ("plot(Signals) 1-32"=→"RefCal 97 - 112":T27, "plot(Signals) 33-64"=→"RefCal 113 - 128":T28)  [unwired: 9 in]
      n330 = call "Cal(SubVI)-2013.vi"("Array"=w451, "dt"=w568, "StartChan"=64 ("ChanStart"), "tstart"=w569, "FitData"=w387) -> ("plot(Signals) 1-32"=→"RefCal 65 - 80":T27, "plot(Signals) 33-64"=→"RefCal 81 - 96":T28)  [unwired: 9 in]
      n331 = Divide(x=w424, y=sgl -1000.0 ("Scale(mV)")) -> (x/y=w389:sgl)
      "T-Start [for Display)\nShould be -1 [s]" <- w389
      n332 = Array Subset(array=w378, index (row)=0, length (row)=64, index (col)=0) -> (w411:sgl[][])  [unwired: 1 in]
      n333 = Array Subset(array=w377, index (row)=0, length (row)=64, index (col)=0) -> (w539:sgl[][])  [unwired: 1 in]
      n334 = Array Subset(array=w378, index (row)=0 ("index"), length (row)=128 ("length")) -> (w415:sgl[][])  [unwired: 2 in]
      n335 = Array Subset(array=w378, index (row)=64, length (row)=64, index (col)=0) -> (w416:sgl[][])  [unwired: 1 in]
      n336 = Compound Arithmetic op=OR(w585, w586, w587) -> (w602:bool[])
      n337 = Array Subset(array=w377, index (row)=64, length (row)=64, index (col)=0) -> (w535:sgl[][])  [unwired: 1 in]
      n338 = Array Subset(array=w377, index (row)=0 ("index"), length (row)=128 ("length")) -> (w374:sgl[][])  [unwired: 2 in]
      n339 = call "Visualize_Signals64.vi"("FPGSampleTime"=w383, "tstart"=w389, "Signals"=w535) -> ("plot(Signals) 33-64"=→"Pow 97 - 128":T26, "plot(Signals) 1-32"=→"Pow 65 - 96":T4)  [unwired: 7 in]
      n340 = call "Visualize_Signals64.vi"("FPGSampleTime"=w383, "tstart"=w389, "Signals"=w539) -> ("plot(Signals) 33-64"=→"Pow 33-64":T26, "plot(Signals) 1-32"=→"Pow 1-32":T4)  [unwired: 7 in]
      n341 = call "Visualize_Signals64.vi"("FPGSampleTime"=w383, "tstart"=w389, "Signals"=w416) -> ("plot(Signals) 33-64"=→"Raw 97 - 128":T26, "plot(Signals) 1-32"=→"Raw 65 - 97":T4)  [unwired: 7 in]
      n342 = call "Visualize_Signals64.vi"("FPGSampleTime"=w383, "tstart"=w389, "Signals"=w411) -> ("plot(Signals) 33-64"=→"Raw 33-64":T26, "plot(Signals) 1-32"=→"Raw 1-32":T4)  [unwired: 7 in]
      n343 = disable-structure shown="Disabled" {
        disable-tunnel: w378 -> [w692 _]
        disable-tunnel: w414 -> [w691 _]
        disable-tunnel: w413 -> [w690 _]
        disable-tunnel: w412 -> [w689 _]
        disable-tunnel: w411 -> [w688 _]
        disable-tunnel: w394 -> [w687 _]
        disable-tunnel: w393 -> [w686 _]
        disable-tunnel: w392 -> [w685 _]
        disable-tunnel: w389 -> [w684 _]
        disable-tunnel: w383 -> [w683 _]
        frame Disabled {
          # "Local TDMS Data Storage"
          n344 = call "W7-X-Bolo-TMDS-LOCAL.vi"("Kappa 2"=w690, "ArrayOutput 4"=w691, "ArrayOutput 3"=w689, "Array"=w688, "RawArray"=w692, "Numeric"=w684, "ArrayOutput"=w685, "Kappa"=w686, "ArrayOutput 2"=w687, "SampleTime"=w683) -> ()  [unwired: 5 in, 1 out]
        }
        frame Enabled {
        }
      }
      n345 = Array Subset(array=w602, index=64, length=32) -> (→"RefStatus 65-96":bool[])
      n346 = Array Subset(array=w602, index=96, length=32) -> (→"RefStatus 97-128":bool[])
      n347 = Array Subset(array=w602, index=0, length=32) -> (→"RefStatus 1-32":bool[])
      n348 = Array Subset(array=w602, index=32, length=32) -> (→"RefStatus 33-64":bool[])
      "Fehler READ U+P" <- w403
    }
    frame True {
      n349 = local write "state"("Error->NoRead" ("state")) -> ()
    }
  }
  n350 = xnode "Read/Write Control"("FPGA VI Reference In"=w67) -> ("FPGA VI Reference Out"=w45:refnum<k20>, "SampleTrigger2"=w68:u32)  [unwired: 1 in, 1 out]
  n351 = To Quad Integer(1:w68) -> (0:w41:i64)
  "Presamples \n(If -1, then no trigger detected)" <- w41
  n352 = Multiply(x=w23, y=w46) -> (x*y=w24:i64)
  n353 = flat-sequence {
    tunnel: w1 -> [w916]
    tunnel: w202 -> [w917]
    tunnel: w45 -> [w918]
    tunnel: [w918] -> w44
    tunnel: [w917] -> w43
    tunnel: [w916] -> w42
    tunnel: w24 -> [w915]
    tunnel: w41 -> [w914]
    tunnel: [w913] -> w40
    tunnel: [w931] -> w39
    tunnel: [w930] -> w38
    tunnel: [w929] -> w37
    tunnel: w44 -> [w931]
    tunnel: w43 -> [w930]
    tunnel: w42 -> [w929]
    tunnel: w39 -> [w938]
    tunnel: [w938] -> w36
    tunnel: w38 -> [w937]
    tunnel: [w937] -> w34
    tunnel: w37 -> [w936]
    tunnel: [w936] -> w32
    tunnel: [w934] -> w2
    tunnel: w36 -> [w945]
    tunnel: [w945] -> w35
    tunnel: w34 -> [w944]
    tunnel: [w944] -> w33
    tunnel: w32 -> [w943]
    tunnel: [w943] -> w31
    tunnel: w35 -> [w951]
    tunnel: w33 -> [w949]
    tunnel: w31 -> [w946]
    frame #0 {
      n354 = case "Correct timebase depending on if Trigger detected" shown="4294967295" w914 {
        selector: w914 -> [w921 _]
        tunnel: [w922 w924] -> w913
        tunnel: w915 -> [w920 _]
        frame Default {
          # "1 Trigger nur während OP"
          # "4294967295"
          # "Trigger deviation [ns]"
          # "Input Sample Frequency"
          n355 = Multiply(x=w921, y=w920) -> (x*y=w919:i64)
          n356 = To Quad Integer(1:w919) -> (0:w922:i64)
        }
        frame 4294967295 {
          # "ms to ns conversion"
          # "4294967295\n=default if not Trigger"
          n357 = local read "DAQ wait time (should be = TWT"() -> (w923:i32)
          n358 = Multiply(x=i64 1000000, y=w923) -> (x*y=w924:i64)
        }
      }
    }
    frame #1 {
      n359 = control-ref of="DAQ Timer"() -> (w926:refnum<vi>)
      n360 = call "W7X-Bolo-Timer.vi"("Wait-Time until Trigger\npublished on CODA\ntypically 10 s"="Wait-Time until Trigger\npublished on CODA\ntypically 10 s", "Digital in"=w926) -> ()  [unwired: 10 in]
      n361 = local write "state"("Wait for published Shot Time (10s)" ("state")) -> ()
    }
    frame #2 {
      n362 = local write "state"("Reading Trigger Time" ("state")) -> ()
      n363 = case shown="1, Default" "Trigger Source" {
        tunnel: [w939 w941 "Set Manual Time [ns]"] -> w934
        tunnel: "Trigger No Choice\nfrom MDS+ Website\n0 for old\n1 during OP" -> [_ w940 _]
        frame 0 {
          n364 = call "Get UTC from NTP.vi"() -> ("UTC Time"=w939:i64)  [unwired: 10 in, 1 out]
        }
        frame 1, Default {
          n365 = call "GetTriggerTime.vi"("TriggerIndex (1)"=w940) -> ("TriggerTime [ns]"=w941:i64)  [unwired: 9 in, 1 out]
        }
        frame 2 {
        }
      }
    }
    frame #3 {
    }
    frame #4 {
      n366 = case shown="True" w946 {
        tunnel: w951 -> [w952 w954]
        tunnel: w949 -> [_ w953]
        tunnel: [w952 _] -> w948
        frame False {
        }
        frame True {
          n367 = xnode "Close FPGA VI Reference"("FPGA VI Reference In"=w954, "error in"=w953) -> ()  [unwired: 1 out]
        }
      }
      "FPGA VI Reference Out" <- w948
      n368 = property on="stop" class="Bool (strict)"("Val(Sgnl)"=TRUE) -> ()  [unwired: 2 in, 2 out]
      n369 = local write "state"("Idle / Waiting for new Trigger" ("state")) -> ()
    }
  }
  n370 = Multiply(x=w24, y=w29) -> (x*y=w28:i64)
  n371 = Initialize Array(w2, w50) -> (w144:i64[])
  n372 = local read "No. of Samples:"() -> (w18:u32)
  n373 = Add(x=w2, y=w40) -> (x+y=w51:i64)
  n374 = for {
    N: w50 -> [_]
    shift-right: [w959] -> w63
    shift-left: w144 -> [w960]
    shift-right: [w956] -> _
    shift-left: w51 -> [w957]
    tunnel: w28 -> [w955]
    i -> [w958]
    n375 = Add(x=w957, y=w955) -> (x+y=w956:i64)
    n376 = Replace Array Subset(array=w960, new element=w957, index=w958) -> (w959:i64[])
  }
  n377 = call "Array_Trans.vi"("RB01"=w131, "Array 8"=w30, "Kappa 2"=w129, "RB01 2"=w132, "Tau 2"=w130, "Kappa"=w71, "Tau"=w72) -> ("Array 7"=w125:dbl[][], "Array 4"=w120:dbl[][], "Array"=w115:dbl[][], "Array 3"=w118:dbl[][], "Array 6"=w124:dbl[][], "Array 2"=w116:dbl[][], "Array 5"=w122:dbl[][])  [unwired: 2 in]
  n378 = To Quad Integer(1:w51) -> (0:w175:i64)
  n379 = Initialize Array(w51, w18) -> (w145:i64[])
  n380 = Build Array(w51) -> (w73:i64[])
  n381 = for {
    N: w18 -> [_]
    shift-right: [w965] -> w17
    shift-left: w145 -> [w966]
    shift-right: [w962] -> _
    shift-left: w51 -> [w963]
    tunnel: w28 -> [w961]
    i -> [w964]
    n382 = Add(x=w963, y=w961) -> (x+y=w962:i64)
    n383 = Replace Array Subset(array=w966, new element=w963, index=w964) -> (w965:i64[])
  }
  n384 = call "W7X2DJSON.vi"("values"=w124, "label"=w96, "dimensionSize"=w76, "dimensions"=w73, "dimensionCount"=128, "sampleCount"=w76, "datatype"=w133) -> ("JSON string"=w95:string)  [unwired: 4 in]
  n385 = call "W7X2DJSON.vi"("values"=w122, "label"=w93, "dimensionSize"=w121, "dimensions"=w73, "dimensionCount"=128, "sampleCount"=w121, "datatype"=w135) -> ("JSON string"=w92:string)  [unwired: 4 in]
  n386 = call "W7X2DJSON.vi"("values"=w125, "label"=w99, "dimensionSize"=w49, "dimensions"=w73, "dimensionCount"=128, "sampleCount"=w49, "datatype"=w127) -> ("JSON string"=w98:string)  [unwired: 4 in]
  n387 = call "W7X2DJSON.vi"("values"=w120, "label"=w90, "dimensionSize"=w119, "dimensions"=w73, "dimensionCount"=128, "sampleCount"=w119, "datatype"=w137) -> ("JSON string"=w89:string)  [unwired: 4 in]
  n388 = call "W7X2DJSON.vi"("values"=w115, "label"=w80, "dimensionSize"=w78, "dimensions"=w73, "dimensionCount"=128, "sampleCount"=w78, "datatype"=w143) -> ("JSON string"=w79:string)  [unwired: 4 in]
  n389 = Replace Array Subset(array=i64[] [1399090569999999999, -1] ("dimensions"), new element=w175, index=0) -> (w13:i64[])
  n390 = call "W7X2DJSON.vi"("values"=w118, "label"=w87, "dimensionSize"=w117, "dimensions"=w73, "dimensionCount"=128, "sampleCount"=w117, "datatype"=w139) -> ("JSON string"=w86:string)  [unwired: 4 in]
  n391 = call <vilib>:"OpenHandle.vi"() -> ("client handle out"=w172:T29, "error out"=w171:errorcluster)  [unwired: 14 in]
  n392 = call "W7X1DPut.vi"("dimensions"=w13, "Unit"=w94, "SigJSONbuffer"=w95, "SigLabel"=w96) -> ()  [unwired: 8 in]
  n393 = call "W7X1DPut.vi"("dimensions"=w13, "Unit"=w88, "SigJSONbuffer"=w89, "SigLabel"=w90) -> ()  [unwired: 8 in]
  n394 = call "W7X1DPut.vi"("dimensions"=w13, "Unit"=w81, "SigJSONbuffer"=w79, "SigLabel"=w80) -> ()  [unwired: 8 in]
  n395 = call "W7X1DPut.vi"("dimensions"=w13, "Unit"=w91, "SigJSONbuffer"=w92, "SigLabel"=w93) -> ()  [unwired: 8 in]
  n396 = call "W7X2DJSON.vi"("values"=w116, "label"=w83, "dimensionSize"=w77, "dimensions"=w73, "dimensionCount"=128, "sampleCount"=w77, "datatype"=w141) -> ("JSON string"=w82:string)  [unwired: 4 in]
  n397 = call "chanDescQSB.vi"("dimensions"=w13, "values"=T19 [{"chanDescs"=[{"name"="E_Chan_1", "active"=1}, {"name"="E_Chan_2", "active"=1}, {"name"="E_Chan_3", "active"=1}, {"name"="E_Chan_4", "active"=1}, {"name"="E_Chan_5", "active"=1}, {"name"="E_Chan_6", "active"=1}, {"name"="E_Chan_7", "active"=1}, {"name"="E_Chan_8", "active"=1}, {"name"="E_Chan_9", "active"=1}, {"name"="E_Chan_10", "active"=1}, {"name"="E_Chan_11", "active"=1}, {"name"="E_Chan_12", "active"=1}, {"name"="E_Chan_13", "active"=1}, {"name"="E_Chan_14", "active"=1}, {"name"="E_Chan_15", "active"=1}, {"name"="E_Chan_16", "active"=1}, {"name"="E_Chan_17", "active"=1}, {"name"="E_Chan_18", "active"=1}, {"name"="E_Chan_19", "active"=1}, {"name"="E_Chan_20", "active"=1}, {"name"="E_Chan_21", "active"=1}, {"name"="E_Chan_22", "active"=1}, {"name"="E_Chan_23", "active"=1}, {"name"="E_Chan_24", "active"=1}, {"name"="E_Chan_25", "active"=1}, {"name"="E_Chan_26", "active"=1}, {"name"="E_Chan_27", "active"=1}, {"name"="E_Chan_28", "active"=1}, {"name"="E_Chan_29", "active"=1}, {"name"="E_Chan_30", "active"=1}, {"name"="E_Chan_31", "active"=1}, {"name"="E_Chan_32", "active"=1}, {"name"="E_Chan_33", "active"=1}, {"name"="E_Chan_34", "active"=1}, {"name"="E_Chan_35", "active"=1}, {"name"="E_Chan_36", "active"=1}, {"name"="E_Chan_37", "active"=1}, {"name"="E_Chan_38", "active"=1}, {"name"="E_Chan_39", "active"=1}, {"name"="E_Chan_40", "active"=1}, {"name"="E_Chan_41", "active"=1}, {"name"="E_Chan_42", "active"=1}, {"name"="E_Chan_43", "active"=1}, {"name"="E_Chan_44", "active"=1}, {"name"="E_Chan_45", "active"=1}, {"name"="E_Chan_46", "active"=1}, {"name"="E_Chan_47", "active"=1}, {"name"="E_Chan_48", "active"=1}, {"name"="E_Chan_49", "active"=1}, {"name"="E_Chan_50", "active"=1}, {"name"="E_Chan_51", "active"=1}, {"name"="E_Chan_52", "active"=1}, {"name"="E_Chan_53", "active"=1}, {"name"="E_Chan_54", "active"=1}, {"name"="E_Chan_55", "active"=1}, {"name"="E_Chan_56", "active"=1}, {"name"="E_Chan_57", "active"=1}, {"name"="E_Chan_58", "active"=1}, {"name"="E_Chan_59", "active"=1}, {"name"="E_Chan_60", "active"=1}, {"name"="E_Chan_61", "active"=1}, {"name"="E_Chan_62", "active"=1}, {"name"="E_Chan_63", "active"=1}, {"name"="E_Chan_64", "active"=1}, {"name"="E_Chan_65", "active"=1}, {"name"="E_Chan_66", "active"=1}, {"name"="E_Chan_67", "active"=1}, {"name"="E_Chan_68", "active"=1}, {"name"="E_Chan_69", "active"=1}, {"name"="E_Chan_70", "active"=1}, {"name"="E_Chan_71", "active"=1}, {"name"="E_Chan_72", "active"=1}, {"name"="E_Chan_73", "active"=1}, {"name"="E_Chan_74", "active"=1}, {"name"="E_Chan_75", "active"=1}, {"name"="E_Chan_76", "active"=1}, {"name"="E_Chan_77", "active"=1}, {"name"="E_Chan_78", "active"=1}, {"name"="E_Chan_79", "active"=1}, {"name"="E_Chan_80", "active"=1}, {"name"="E_Chan_81", "active"=1}, {"name"="E_Chan_82", "active"=1}, {"name"="E_Chan_83", "active"=1}, {"name"="E_Chan_84", "active"=1}, {"name"="E_Chan_85", "active"=1}, {"name"="E_Chan_86", "active"=1}, {"name"="E_Chan_87", "active"=1}, {"name"="E_Chan_88", "active"=1}, {"name"="E_Chan_89", "active"=1}, {"name"="E_Chan_90", "active"=1}, {"name"="E_Chan_91", "active"=1}, {"name"="E_Chan_92", "active"=1}, {"name"="E_Chan_93", "active"=1}, {"name"="E_Chan_94", "active"=1}, {"name"="E_Chan_95", "active"=1}, {"name"="E_Chan_96", "active"=1}, {"name"="E_Chan_97", "active"=1}, {"name"="E_Chan_98", "active"=1}, {"name"="E_Chan_99", "active"=1}, {"name"="E_Chan_100", "active"=1}, {"name"="E_Chan_101", "active"=1}, {"name"="E_Chan_102", "active"=1}, {"name"="E_Chan_103", "active"=1}, {"name"="E_Chan_104", "active"=1}, {"name"="E_Chan_105", "active"=1}, {"name"="E_Chan_106", "active"=1}, {"name"="E_Chan_107", "active"=1}, {"name"="E_Chan_108", "active"=1}, {"name"="E_Chan_109", "active"=1}, {"name"="E_Chan_110", "active"=1}, {"name"="E_Chan_111", "active"=1}, {"name"="E_Chan_112", "active"=1}, {"name"="E_Chan_113", "active"=1}, {"name"="E_Chan_114", "active"=1}, {"name"="E_Chan_115", "active"=1}, {"name"="E_Chan_116", "active"=1}, {"name"="E_Chan_117", "active"=1}, {"name"="E_Chan_118", "active"=1}, {"name"="E_Chan_119", "active"=1}, {"name"="E_Chan_120", "active"=1}, {"name"="E_Chan_121", "active"=1}, {"name"="E_Chan_122", "active"=1}, {"name"="E_Chan_123", "active"=1}, {"name"="E_Chan_124", "active"=1}, {"name"="E_Chan_125", "active"=1}, {"name"="E_Chan_126", "active"=1}, {"name"="E_Chan_127", "active"=1}, {"name"="E_Chan_128", "active"=1}]}], "label"="parms") -> ()  [unwired: 1 out]
  n398 = call <vilib>:"AddHeader.vi"("client handle"=w172, "header"="Content-Type", "value"="application/json", "error in (no error)"=w171) -> ("client handle out"=w170:T29, "error out"=w169:errorcluster)  [unwired: 10 in]
  n399 = call "parmsQSB.vi"("dimensions"=w13, "values"=T18 [{"Nchannel"=128, "ADCbits"=16, "BridgeVoltage (V)"=5.0, "ExptSampleFrequency (Hz)"=2500.0, "CalibSampleFrequency (Hz)"=2500.0, "CalStep1 (V)"="2.5", "CalStep2 (V)"="3.7", "detector"="Au_Kapton"}], "label"="parms") -> ("JSON string"=w65:string)
  n400 = call "W7X1DPut.vi"("dimensions"=w13, "Unit"=w97, "SigJSONbuffer"=w98, "SigLabel"=w99) -> ()  [unwired: 8 in]
  n401 = call "W7X1DPut.vi"("dimensions"=w13, "Unit"=w85, "SigJSONbuffer"=w86, "SigLabel"=w87) -> ()  [unwired: 8 in]
  n402 = local read "SampleTime"() -> (w10:sgl)
  n403 = local read "SampleTime"() -> (w7:sgl)
  n404 = call "W7X1DPut.vi"("dimensions"=w13, "Unit"=w84, "SigJSONbuffer"=w82, "SigLabel"=w83) -> ()  [unwired: 8 in]
  n405 = Multiply(x=w18, y=w7) -> (x*y=w8:sgl)
  n406 = call-poly <vilib>:"POST.vi"("client handle"=w170, "url"="http://archive-webapi/Test/raw/W7X/QSB_Bolometry/File_PARLOG/", "buffer"=w65, "error in (no error)"=w169, "timeout (10000)"=400000 ("timeout for upload")) -> ("client handle out"=w174:T29, "headers"=→"headers chanDesc":string, "body"=→"body chanDesc":string, "error out"=w60:errorcluster)  [unwired: 7 in]
  n407 = Reciprocal(x=w10) -> (1/x=w52:sgl)
  n408 = Reciprocal(x=w10) -> (1/x=w53:sgl)
  n409 = Reciprocal(x=w7) -> (1/x=w55:sgl)
  n410 = Reciprocal(x=w7) -> (1/x=w59:sgl)
  n411 = Reciprocal(x=w7) -> (1/x=w57:sgl)
  n412 = call "W7X2DJSON.vi"("values"=w21, "label"=w14, "dimensionSize"=w18, "dimensions"=w17, "dimensionCount"=128, "sampleCount"=w18, "datatype"=w20) -> ("JSON string"=w15:string)  [unwired: 4 in]
  n413 = call "W7X2DJSON.vi"("values"=w149, "label"=w104, "dimensionSize"=w160, "dimensions"=w63, "dimensionCount"=128, "sampleCount"=w160, "datatype"=w162) -> ("JSON string"=w103:string)  [unwired: 4 in]
  n414 = call "W7X2DJSON.vi"("values"=w147, "label"=w108, "dimensionSize"=w154, "dimensions"=w63, "dimensionCount"=128, "sampleCount"=w154, "datatype"=w156) -> ("JSON string"=w107:string)  [unwired: 4 in]
  n415 = call "W7X2DJSON.vi"("values"=w148, "label"=w114, "dimensionSize"=w151, "dimensions"=w63, "dimensionCount"=128, "sampleCount"=w151, "datatype"=w153) -> ("JSON string"=w113:string)  [unwired: 4 in]
  n416 = call "W7X2DJSON.vi"("values"=w22, "label"=w101, "dimensionSize"=w18, "dimensions"=w17, "dimensionCount"=128, "sampleCount"=w18, "datatype"=w163) -> ("JSON string"=w100:string)  [unwired: 4 in]
  n417 = call "W7X2DJSON.vi"("values"=w150, "label"=w6, "dimensionSize"=w157, "dimensions"=w63, "dimensionCount"=128, "sampleCount"=w157, "datatype"=w159) -> ("JSON string"=w16:string)  [unwired: 4 in]
  n418 = To Unsigned Word Integer(number=w52) -> (unsigned 16bit integer=w25:u16)
  n419 = To Unsigned Word Integer(number=w53) -> (unsigned 16bit integer=w11:u16)
  n420 = To Unsigned Word Integer(number=w55) -> (unsigned 16bit integer=w54:u16)
  n421 = To Unsigned Word Integer(number=w59) -> (unsigned 16bit integer=w58:u16)
  n422 = To Unsigned Word Integer(number=w57) -> (unsigned 16bit integer=w56:u16)
  n423 = call <vilib>:"CloseHandle.vi"("client handle"=w174, "error in (no error)"=w60) -> ("error out"=w164:errorcluster)  [unwired: 13 in]
  n424 = call "saveToFile.vi"("SigJSONbuffer"=w65, "dimensions"=w63, "String"="File_PARLOG" ("name or relative path")) -> ("error out"=w61:errorcluster)  [unwired: 8 in]
  n425 = call "W7X2DPut.vi"("dimensions"=w13, "pulse_length"=w8, "Unit"=w9, "sample period"=w7, "sample rate"=w11, "SigJSONbuffer"=w15, "SigLabel"=w14) -> ()  [unwired: 4 in, 1 out]
  n426 = Merge Errors(w164, w61) -> (→"parms error out":errorcluster)
  n427 = call "W7X2DPut_DAZ.vi"("dimensions"=w13, "pulse_length"=4.0, "Unit"=w26, "sample period"=w10, "sample rate"=w25, "SigJSONbuffer"=w16, "SigLabel"=w6) -> ()  [unwired: 4 in, 1 out]
  n428 = call "W7X2DPut.vi"("dimensions"=w13, "pulse_length"=4.0, "Unit"=w110, "sample period"=w10, "sample rate"=w11, "SigJSONbuffer"=w107, "SigLabel"=w108) -> ("Parlog error out"=→"Parlog error out  2":errorcluster)  [unwired: 4 in]
  n429 = call "W7X2DPut.vi"("dimensions"=w13, "pulse_length"=w8, "Unit"=w102, "sample period"=w7, "sample rate"=w54, "SigJSONbuffer"=w100, "SigLabel"=w101) -> ()  [unwired: 4 in, 1 out]
  n430 = call "W7X2DPut.vi"("dimensions"=w13, "pulse_length"=4.0, "Unit"=w106, "sample period"=w7, "sample rate"=w58, "SigJSONbuffer"=w103, "SigLabel"=w104) -> ()  [unwired: 4 in, 1 out]
  n431 = call "W7X2DPut.vi"("dimensions"=w13, "pulse_length"=4.0, "Unit"=w112, "sample period"=w10, "sample rate"=w56, "SigJSONbuffer"=w113, "SigLabel"=w114) -> ("Parlog error out"=→"Parlog error out":errorcluster)  [unwired: 4 in]
  "result" <- w4
